vi "2d Flyover.vi"() -> ()   [LabVIEW 2022 SP3]
uses:
  C:/Users/mnopl/OneDrive/Documents/2DFlyover/2D Flyover/Thorlabs.MotionControl.Controls.dll
  Thorlabs.MotionControl.Controls.dll
  Action Engine/ActionEngineEnum.ctl
  <vilib>/DAQmx/read.llb/DAQmx Read (Analog 1D DBL 1Chan NSamp).vi
  <vilib>/Analysis/baseanly.llb/Mean (DBL).vi
  <vilib>/DAQmx/miscellaneous.llb/DAQmx Fill In Error Info.vi
  <vilib>/Analysis/NI_AALBase.lvlib
panel:
  in  "Stop":bool
  in  "Settings Y":T1={"Step Size (mm)"=10.0, "Initial Position"=0.0, "Move Absolute/Relative Position"=0.0, "Step Delay (ms)"=0, "Velocity (mm/s)"=0.0, "Acceleration (mm/s^2)"=0.0} {"Step Size (mm)" min=0.00046 format="%.8f"}
  in  "Settings X":T1={"Step Size (mm)"=10.0, "Initial Position"=0.0, "Move Absolute/Relative Position"=0.0, "Step Delay (ms)"=0, "Velocity (mm/s)"=0.0, "Acceleration (mm/s^2)"=0.0} {"Step Size (mm)" min=0.00046 format="%.8f"}
  in  "Acceleration":dbl=2.0
  in  "Estimate X Step Size":bool
  in  "2D Flyover":bool
  in  "Flyover Y Linescan":bool
  in  "Update Vel/Acc":bool
  in  "Save Line graph":bool
  out "Time Left":dbl
  out "Line Scan":dbl[](graph)
  in  "Move to Saved Pos":bool
  in  "Save Position":bool
  out "Y Pos 1":dbl
  out "X Pos 1":dbl
  in  "Save Data":bool
  in  "Move to Origin":bool
  in  "Measures/Pixel":dbl=5.0
  in  "Flyover X Linescan":bool
  in  "Move Y":bool
  in  "Move X":bool
  in  "Y Step Size":dbl=1.0
  in  "X Step Size":dbl=1.0
  in  "Move to Y":bool
  in  "Move to X":bool
  in  "Y Move":dbl=1.0
  in  "X Move":dbl=1.0
  out "Y Line Scan":dbl[](array[numeric])=[-inf, -inf, -inf, -inf, -inf, -inf]
  out "X Line Scan":dbl[](array[numeric])=[-inf, -inf, -inf, -inf, -inf, -inf]
  out "Y Origin":dbl
  out "X Orign":dbl
  out "Scan Type":string="Scan"
  in  "Y Line Scan":bool
  in  "Abort":bool
  in  "X Line Scan":bool
  out "(X,Y)":cluster{dbl, dbl}[][](array[cluster])
  in  "Save Image":bool
  in  "Move to Cursor":bool
  in  "Y Pos":dbl=0.899996795693412
  in  "X Pos":dbl=1.0
  in  "Read Position":bool
  out "Graph":dbl[][](graph)
  out "array of values":dbl[][](array[numeric])=[[-inf, -inf, -inf, -inf, -inf, -inf], [-inf, -inf, -inf, -inf, -inf, -inf], [-inf, -inf, -inf, -inf, -inf, -inf], [-inf, -inf, -inf, -inf, -inf, -inf], [-inf, -inf, -inf, -inf, -inf, -inf], [-inf, -inf, -inf, -inf, -inf, -inf]]
  out "task out":refnum<k21>
  in  "physical channels":tag="Dev3/ai0"
  in  "number of samples":i32=10000
  in  "rate":dbl=250000.0
  in  "maximum value":dbl=5.0 format="%0.2f"
  in  "minimum value":dbl=-5.0 format="%0.2f"
  out "Done Mov?":bool=TRUE
  in  "Y Length":dbl=5.0
  in  "X Length":dbl=5.0
  in  "2D Scan":bool
  in  "Velocity":dbl=2.0
  in  "Move Y (in)":bool
  in  "Move X (in)":bool
  in  "Y Step Size (in)":dbl=1.0
  in  "X Step Size (in)":dbl=1.0
  in  "X=T,Y=F":bool
  in  "Moving?":bool
  in  "KCubeStepperControl Y":refnum<k24>(container)
  in  "KCubeStepperControl X":refnum<k24>(container)
  in  "SerialNumber X":string="26005327"
  in  "SerialNumber Y":string="26005279"
  in  "Set Vel/Acc":bool
  # "Internal Variables"
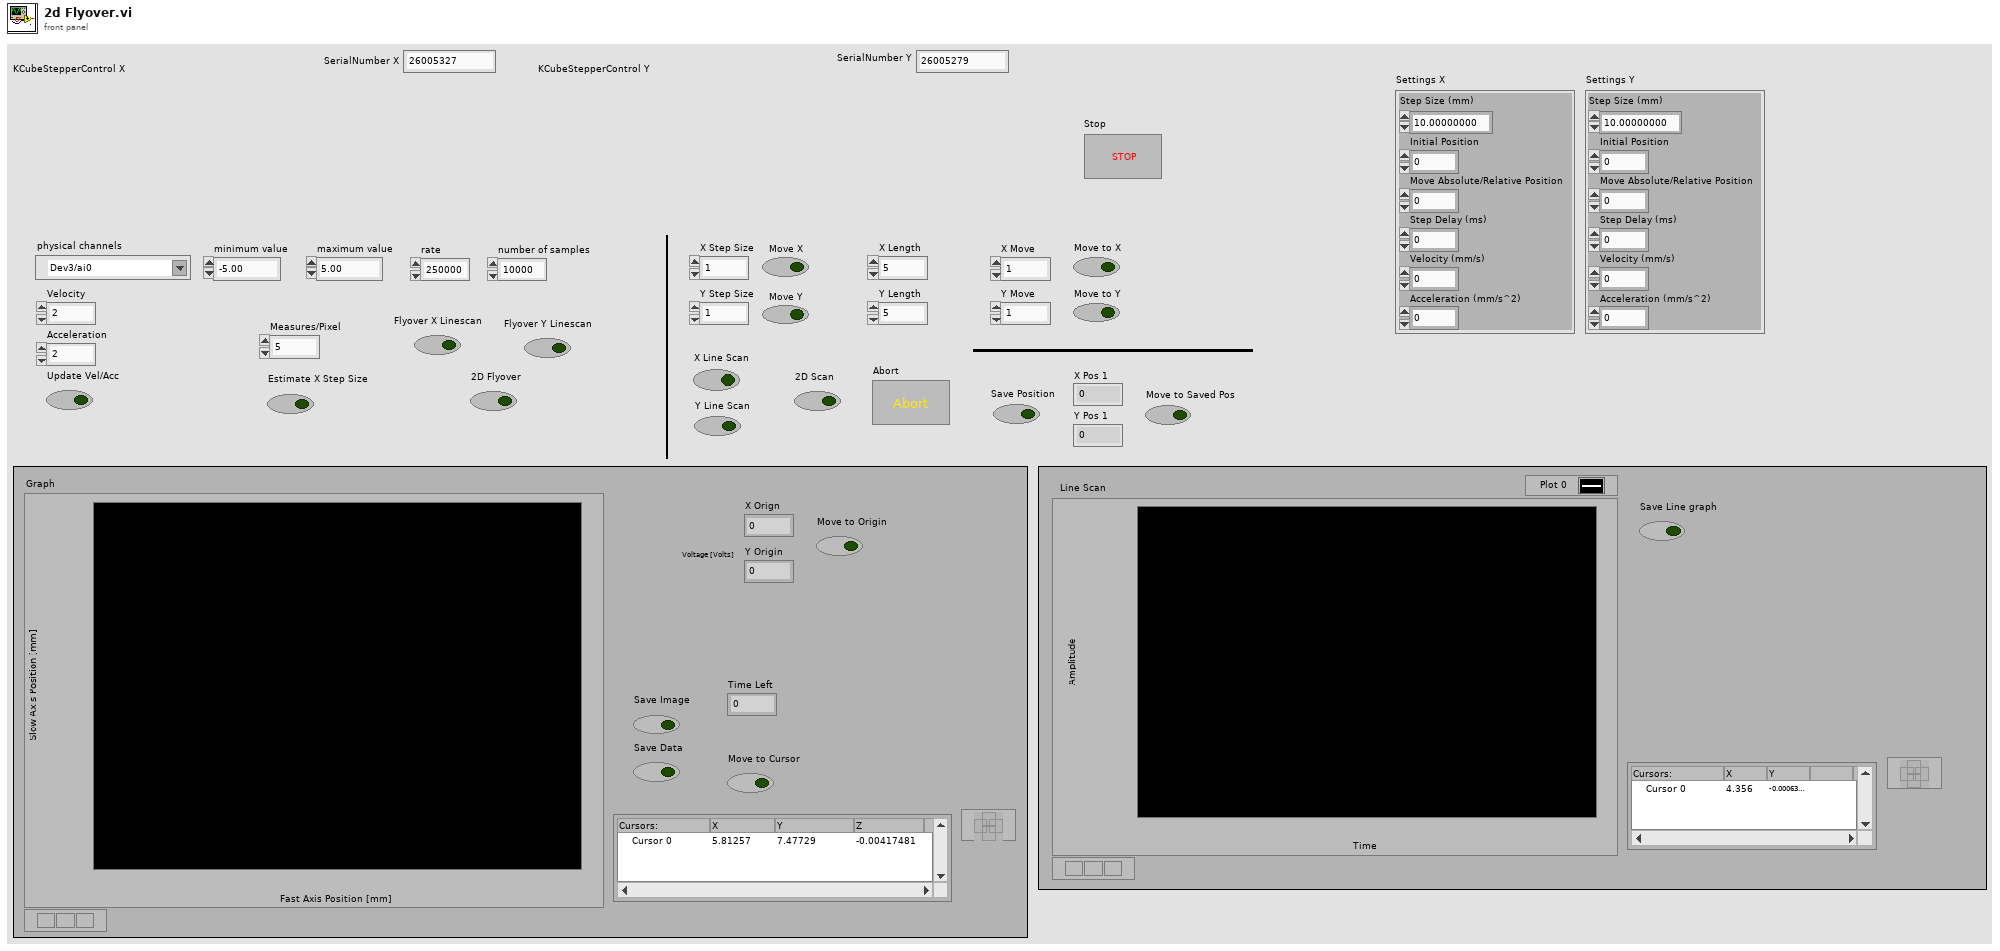
[diagram p1: front panel]
types:
  T1 = cluster{"Step Size (mm)":sgl, "Initial Position":dbl, "Move Absolute/Relative Position":dbl, "Step Delay (ms)":u32, "Velocity (mm/s)":dbl, "Acceleration (mm/s^2)":dbl}
  T2 = typedef "ActionEngineEnum.ctl" = enum16{"Open Connection", "Done", "Get Position", "Settings", "Home", "Move Absolute", "Move Relative", "Step", "Stop Action", "Close Connection"}
  T3 = typedef "LVPointDoubleTypeDef.ctl" = cluster{"Cursor X":dbl, "Cursor Y":dbl}
  T4 = typedef "imagedata.ctl" = cluster{"image type":i32, "image depth":i32, "image":u8[], "mask":u8[], "colors":u32[], "Rectangle":cluster{"left":i16, "top":i16, "right":i16, "bottom":i16}}
  T5 = cluster{"Y Step Size (in)":dbl, "Initial Position":dbl, "Move Absolute/Relative Position":dbl, "Step Delay (ms)":u32, "Velocity (mm/s)":dbl, "Acceleration (mm/s^2)":dbl}
  T6 = cluster{"X Step Size (in)":dbl, "Initial Position":dbl, "Move Absolute/Relative Position":dbl, "Step Delay (ms)":u32, "Velocity (mm/s)":dbl, "Acceleration (mm/s^2)":dbl}
  T7 = cluster{"Step Size (mm)":sgl, "Initial Position":dbl, "Move Absolute/Relative Position":dbl, "Step Delay (ms)":u32, "Velocity":dbl, "Acceleration":dbl}
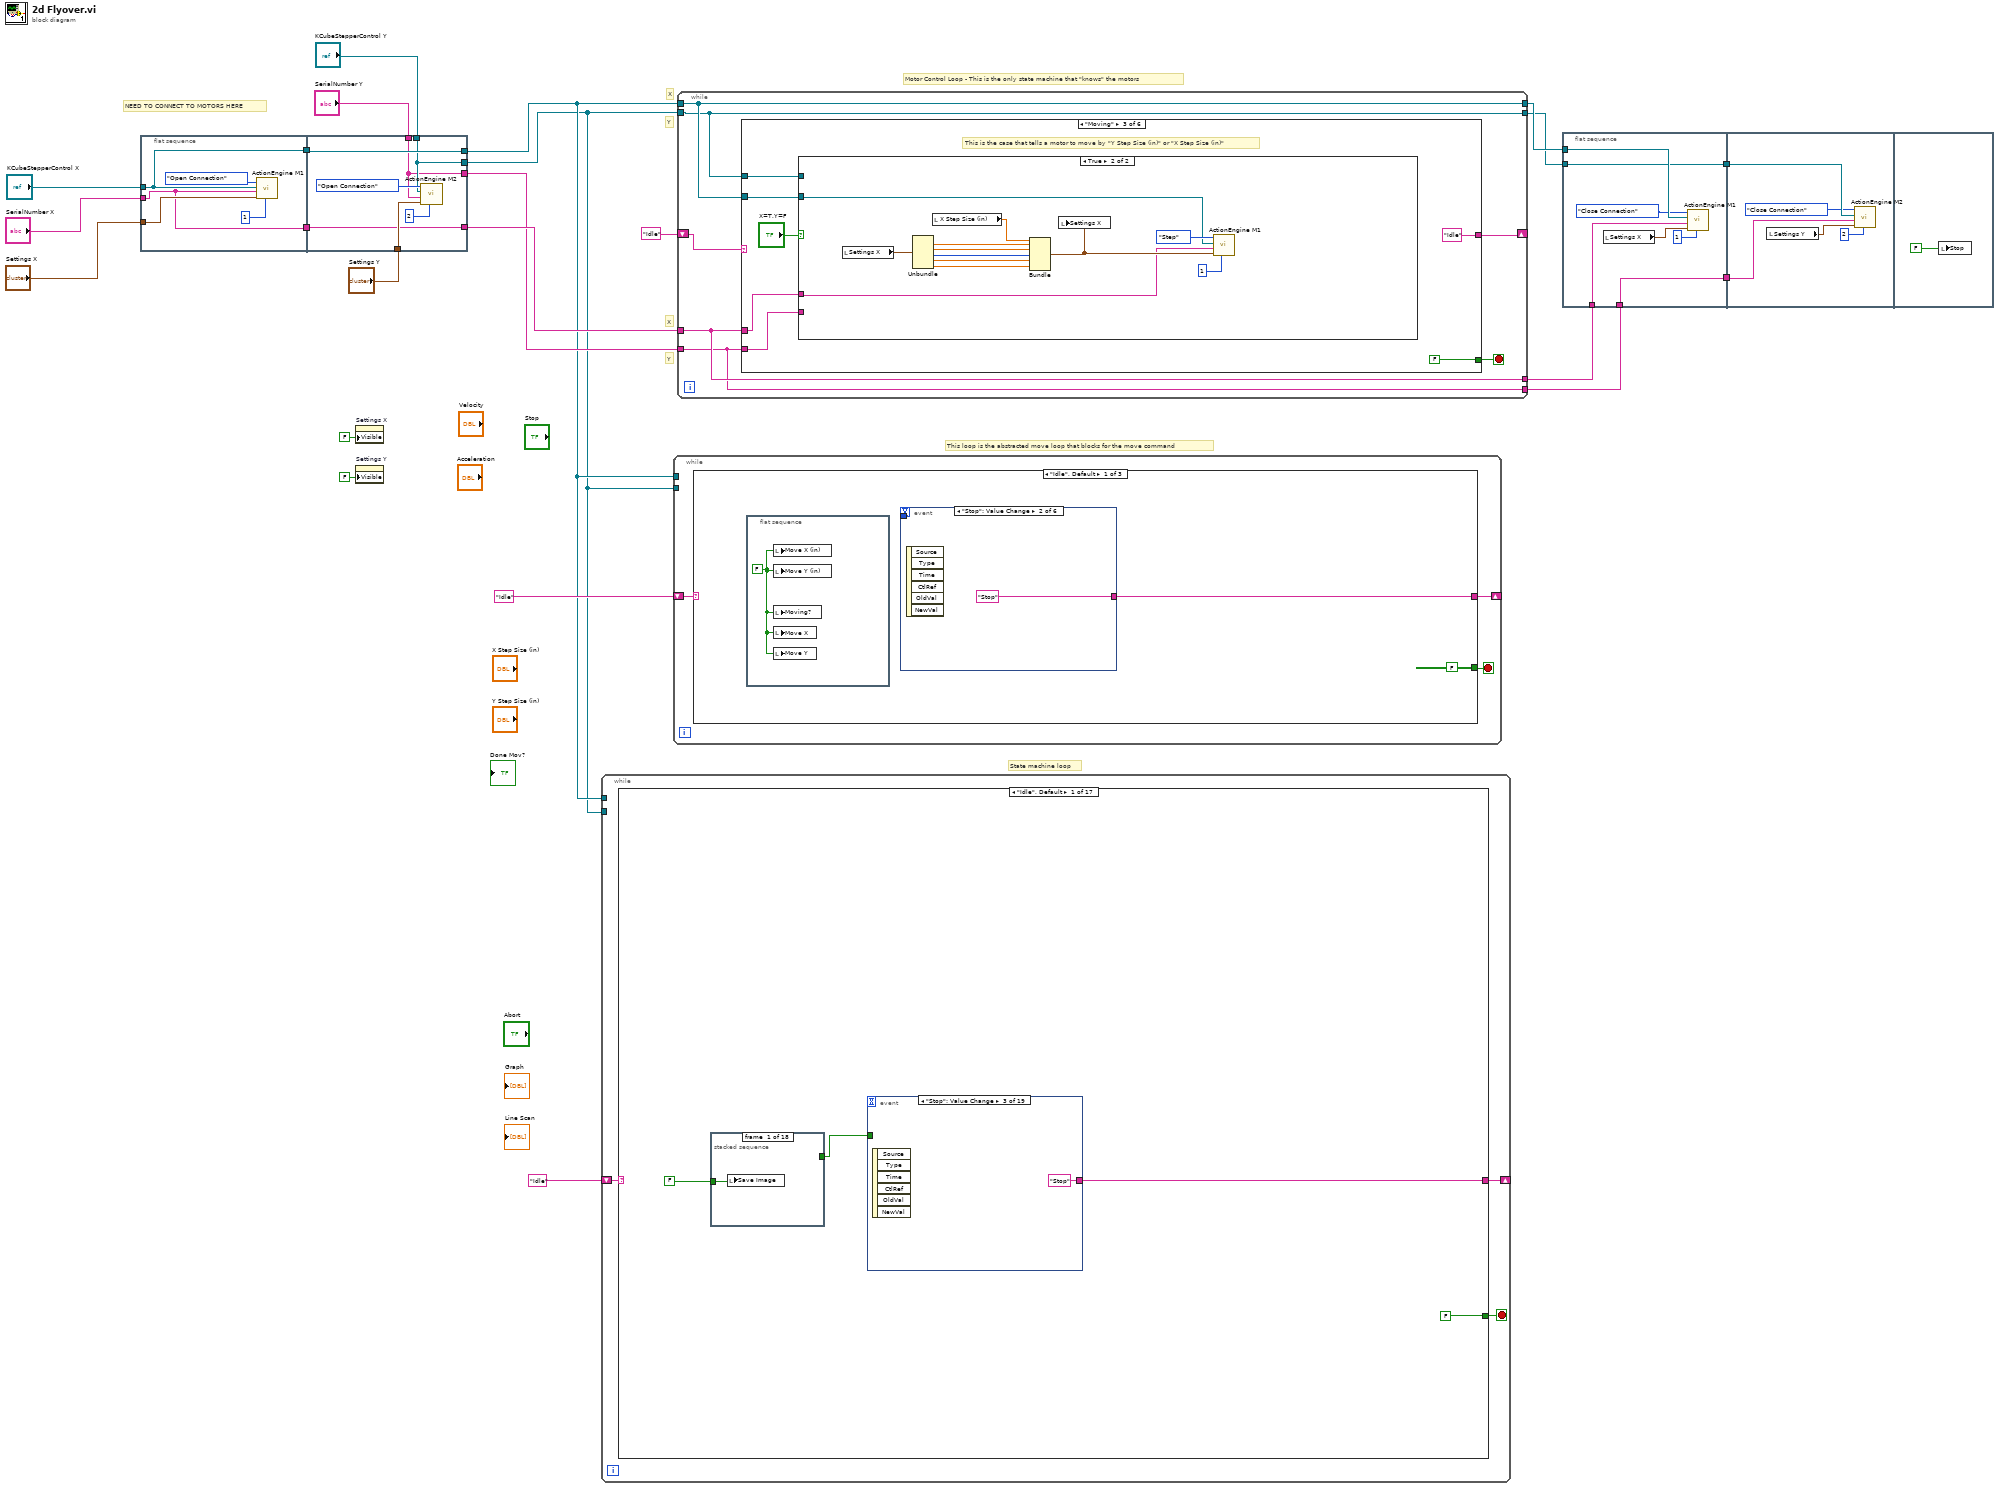
[diagram p0: block diagram]
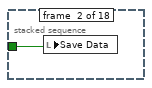
[diagram p2: hidden frame]
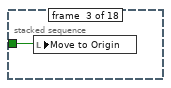
[diagram p3: hidden frame]
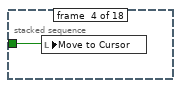
[diagram p4: hidden frame]
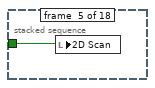
[diagram p5: hidden frame]
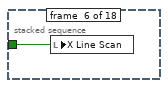
[diagram p6: hidden frame]
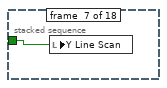
[diagram p7: hidden frame]
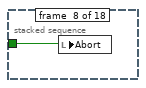
[diagram p8: hidden frame]
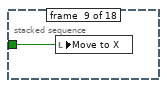
[diagram p9: hidden frame]
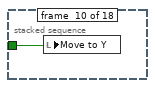
[diagram p10: hidden frame]
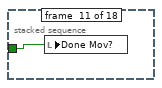
[diagram p11: hidden frame]
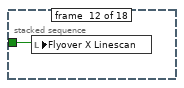
[diagram p12: hidden frame]
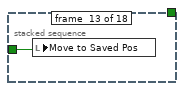
[diagram p13: hidden frame]
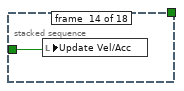
[diagram p14: hidden frame]
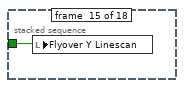
[diagram p15: hidden frame]
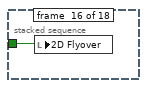
[diagram p16: hidden frame]
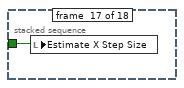
[diagram p17: hidden frame]
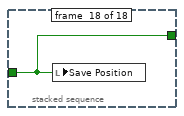
[diagram p18: hidden frame]
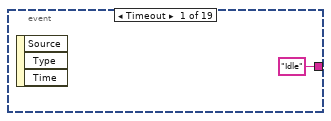
[diagram p19: hidden frame]
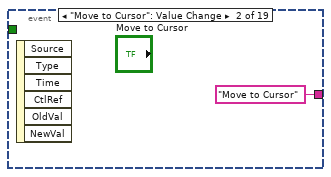
[diagram p20: hidden frame]
diagram:
  # "Y"
  # "X"
  # "NEED TO CONNECT TO MOTORS HERE"
  # "State machine loop"
  # "Y"
  # "X"
  # "This loop is the abstracted move loop that blocks for the move command"
  # "Motor Control Loop - This is the only state machine that \"knows\" the motors"
  n1 = flat-sequence {
    tunnel: "KCubeStepperControl X" -> [w25]
    tunnel: "SerialNumber X" -> [w24]
    tunnel: "Settings X" -> [w26]
    tunnel: [w25] -> w14
    tunnel: [w24] -> w13
    tunnel: "KCubeStepperControl Y" -> [w31]
    tunnel: "SerialNumber Y" -> [w29]
    tunnel: "Settings Y" -> [w33]
    tunnel: w14 -> [w32]
    tunnel: [w32] -> w10
    tunnel: [w31] -> w9
    tunnel: w13 -> [w30]
    tunnel: [w30] -> w12
    tunnel: [w29] -> w11
    frame #0 {
      n2 = call "ActionEngine M1.vi"("ChannelNumber"=1, "Settings"=w26, "SerialNumber"=w24, "KCubeStepperControl"=w25, "Action"=ActionEngineEnum."Open Connection") -> ()  [unwired: 4 in, 2 out]
    }
    frame #1 {
      n3 = call "ActionEngine M2.vi"("ChannelNumber"=2, "Settings"=w33, "SerialNumber"=w29, "KCubeStepperControl"=w31, "Action"=ActionEngineEnum."Open Connection") -> ()  [unwired: 4 in, 2 out]
    }
  }
  n4 = property on="Settings X" class="Clust (strict)"("Visible"=FALSE) -> ()  [unwired: 2 in, 2 out]
  n5 = property on="Settings Y" class="Clust (strict)"("Visible"=FALSE) -> ()  [unwired: 2 in, 2 out]
  n6 = while {
    shift-right: [w37] -> _
    shift-left: "Idle" -> [w38]
    tunnel: w10 -> [_]
    tunnel: w9 -> [_]
    stop <- w36 stop-if-true
    n7 = case shown="\"Idle\", Default" w38 {
      tunnel: [w42 "Init Graph" w132 "Move to Origin" w471 "Idle" ("Scan Type") "Move to Origin" ("Scan Type") "Move to Origin" ("Scan Type") "Idle" ("Scan Type") "Idle" ("Scan Type") "Idle" "Idle" ("Scan Type") "Idle" ("Scan Type") "Idle" ("Scan Type") "Idle" "Idle" ("Scan Type") "Idle"] -> w37
      tunnel: [FALSE FALSE FALSE FALSE FALSE FALSE FALSE FALSE FALSE FALSE FALSE FALSE FALSE FALSE FALSE FALSE TRUE] -> w36
      frame "Idle", Default {
        n8 = stacked-sequence {
          tunnel: FALSE -> [w43 w44 w45 w46 w47 w48 w49 w50 w51 w52 w53 w54 w55 w56 w57 w58 w59 w60]
          tunnel: [_ _ _ _ _ _ _ _ _ _ _ _ _ _ _ _ _ w60] -> w39
          frame #0 {
            n9 = local write "Save Image"(w43) -> ()
          }
          frame #1 {
            n10 = local write "Save Data"(w44) -> ()
          }
          frame #2 {
            n11 = local write "Move to Origin"(w45) -> ()
          }
          frame #3 {
            n12 = local write "Move to Cursor"(w46) -> ()
          }
          frame #4 {
            n13 = local write "2D Scan"(w47) -> ()
          }
          frame #5 {
            n14 = local write "X Line Scan"(w48) -> ()
          }
          frame #6 {
            n15 = local write "Y Line Scan"(w49) -> ()
          }
          frame #7 {
            n16 = local write "Abort"(w50) -> ()
          }
          frame #8 {
            n17 = local write "Move to X"(w51) -> ()
          }
          frame #9 {
            n18 = local write "Move to Y"(w52) -> ()
          }
          frame #10 {
            n19 = local write "Done Mov?"(w53) -> ()
          }
          frame #11 {
            n20 = local write "Flyover X Linescan"(w54) -> ()
          }
          frame #12 {
            n21 = local write "Move to Saved Pos"(w55) -> ()
          }
          frame #13 {
            n22 = local write "Update Vel/Acc"(w56) -> ()
          }
          frame #14 {
            n23 = local write "Flyover Y Linescan"(w57) -> ()
          }
          frame #15 {
            n24 = local write "2D Flyover"(w58) -> ()
          }
          frame #16 {
            n25 = local write "Estimate X Step Size"(w59) -> ()
          }
          frame #17 {
            n26 = local write "Save Position"(w60) -> ()
          }
        }
        n27 = event shown="[2] \"Stop\": Value Change" {
          selector: _ -> [_ _ _ _ _ _ _ _ _ _ _ _ _ _ _ _ _ _ _]
          dyn-events: _ -> [_ _ _ _ _ _ _ _ _ _ _ _ _ _ _ _ _ _ _]
          timeout: _ -> [_ _ _ _ _ _ _ _ _ _ _ _ _ _ _ _ _ _ _]
          tunnel: ["Idle" "Move to Cursor" "Stop" "Init Daq" "Init Daq" "Move to Origin" "Move to Saved Position" "Init Daq" "Init Daq" "Init Daq" "Init Daq" "Move to" "Move to" "Update Vel/Acc" "Save Position" "Save Image" "Save Line graph" "Save Data" "Estimate X Step Size"] -> w42
          tunnel: w39 -> [_ _ _ _ _ _ _ _ _ _ _ _ _ _ _ _ _ _ _]
          event Timeout {
            n28 = event-data() -> ()  [unwired: 1 in, 3 out]
          }
          event "Move to Cursor": Value Change {
            n29 = event-data() -> ()  [unwired: 1 in, 6 out]
          }
          event "Stop": Value Change {
            n30 = event-data() -> ()  [unwired: 1 in, 6 out]
          }
          event "2D Scan": Value Change {
            n31 = event-data() -> ()  [unwired: 1 in, 6 out]
            n32 = local read "X Step Size"() -> (w64:dbl)
            n33 = local read "Y Step Size"() -> (w65:dbl)
            n34 = local write "Scan Type"("Scan" ("Scan Type")) -> ()
            n35 = local write "Y Step Size (in)"(w65) -> ()
            n36 = local write "X Step Size (in)"(w64) -> ()
          }
          event "2D Flyover": Value Change {
            n37 = event-data() -> ()  [unwired: 1 in, 6 out]
            n38 = local read "Y Step Size"() -> (w69:dbl)
            n39 = local read "X Step Size"() -> (w70:dbl)
            n40 = local write "X Step Size (in)"(w70) -> ()
            n41 = local write "Y Step Size (in)"(w69) -> ()
            n42 = local write "Scan Type"("Flyover Scan" ("Scan Type")) -> ()
          }
          event "Move to Origin": Value Change {
            n43 = event-data() -> ()  [unwired: 1 in, 6 out]
          }
          event "Move to Saved Pos": Value Change {
            n44 = event-data() -> ()  [unwired: 1 in, 6 out]
          }
          event "X Line Scan": Value Change {
            n45 = event-data() -> ()  [unwired: 1 in, 6 out]
            n46 = local read "X Step Size"() -> (w74:dbl)
            n47 = local write "X Step Size (in)"(w74) -> ()
            n48 = local write "Scan Type"("Line Scan" ("Scan Type")) -> ()
            n49 = local write "X=T,Y=F"(TRUE ("X=T,Y=F")) -> ()
          }
          event "Flyover X Linescan": Value Change {
            n50 = event-data() -> ()  [unwired: 1 in, 6 out]
            n51 = local read "X Step Size"() -> (w81:dbl)
            n52 = local write "X Step Size (in)"(w81) -> ()
            n53 = local write "Scan Type"("Flyover Linescan" ("Scan Type")) -> ()
            n54 = local write "X=T,Y=F"(TRUE ("X=T,Y=F")) -> ()
          }
          event "Flyover Y Linescan": Value Change {
            n55 = event-data() -> ()  [unwired: 1 in, 6 out]
            n56 = local read "Y Step Size"() -> (w83:dbl)
            n57 = local write "Y Step Size (in)"(w83) -> ()
            n58 = local write "Scan Type"("Flyover Linescan" ("Scan Type")) -> ()
            n59 = local write "X=T,Y=F"(FALSE ("X=T,Y=F")) -> ()
          }
          event "Y Line Scan": Value Change {
            n60 = event-data() -> ()  [unwired: 1 in, 6 out]
            n61 = local read "Y Step Size"() -> (w86:dbl)
            n62 = local write "Y Step Size (in)"(w86) -> ()
            n63 = local write "X=T,Y=F"(FALSE ("X=T,Y=F")) -> ()
            "Scan Type" <- "Line Scan" ("Scan Type")
          }
          event "Move to X": Value Change {
            n64 = event-data() -> ()  [unwired: 1 in, 6 out]
            n65 = local write "X=T,Y=F"(TRUE ("X=T,Y=F")) -> ()
          }
          event "Move to Y": Value Change {
            n66 = event-data() -> ()  [unwired: 1 in, 6 out]
            n67 = local write "X=T,Y=F"(FALSE ("X=T,Y=F")) -> ()
          }
          event "Update Vel/Acc": Value Change {
            n68 = event-data() -> ()  [unwired: 1 in, 6 out]
          }
          event "Save Position": Value Change {
            n69 = event-data() -> ()  [unwired: 1 in, 6 out]
          }
          event "Save Image": Value Change {
            n70 = event-data() -> ()  [unwired: 1 in, 6 out]
          }
          event "Save Line graph": Value Change {
            n71 = event-data() -> ()  [unwired: 1 in, 6 out]
          }
          event "Save Data": Value Change {
            n72 = event-data() -> ()  [unwired: 1 in, 6 out]
          }
          event "Estimate X Step Size": Value Change {
            n73 = event-data() -> ()  [unwired: 1 in, 6 out]
          }
        }
      }
      frame "Init Daq" {
        w100 = -inf
        n74 = local read "Y Length"() -> (w113:dbl)
        n75 = local read "Y Step Size"() -> (w112:dbl)
        n76 = local read "X Length"() -> (w110:dbl)
        n77 = local read "X Step Size"() -> (w109:dbl)
        n78 = Divide(x=w113, y=w112) -> (x/y=w114:dbl)
        n79 = Divide(x=w110, y=w109) -> (x/y=w111:dbl)
        n80 = Round Toward +Infinity(x=w114) -> (ceil(x): smallest int >= x=w103:dbl)
        n81 = Round Toward +Infinity(x=w111) -> (ceil(x): smallest int >= x=w108:dbl)
        n82 = Increment(x=w103) -> (x+1=w101:dbl)
        n83 = Increment(x=w108) -> (x+1=w102:dbl)
        n84 = call "Initialize DAQ Assistant.vi"("minimum value"="minimum value", "maximum value"="maximum value", "rate"="rate", "number of samples"="number of samples", "physical channels"="physical channels") -> ("task out"=→"task out":refnum<k21>)  [unwired: 5 in, 1 out]
        n85 = Initialize Array(w100, w101) -> (→"Y Line Scan":dbl[])
        n86 = Initialize Array(w100, w102, w101) -> (→"array of values":dbl[][])
        n87 = Initialize Array(w100, w102) -> (→"X Line Scan":dbl[])
      }
      frame "Init Graph" {
        n88 = local read "Acceleration"() -> (w128:dbl)
        n89 = local read "Scan Type"() -> (w132:string)
        n90 = local read "Velocity"() -> (w129:dbl)
        n91 = flat-sequence {
          tunnel: [w201] -> w122
          tunnel: ["X Pos"] -> w134
          tunnel: ["Y Pos"] -> w133
          frame #0 {
            n92 = property on="Read Position" class="Bool (strict)"("Val(Sgnl)"=TRUE) -> ()  [unwired: 2 in, 2 out]
          }
          frame #1 {
            n93 = while {
              tunnel: [w202] -> w201
              stop <- w205 stop-if-true
              n94 = local read "Read Position"() -> (w204:bool)
              n95 = Not(x=w204) -> (.not. x?=w205:bool)
              n96 = Wait (ms)(milliseconds to wait=u32 10) -> (millisecond timer value=w202:u32)
            }
          }
          frame #2 {
            "X Orign" <- "X Pos"
            "Y Origin" <- "Y Pos"
          }
        }
        n97 = case shown="\"Line Scan\", Default" w132 {
          tunnel: [w150 w168 w184] -> w126
          tunnel: w125 -> [w150 w168 w184]
          frame "Line Scan", Default {
            n98 = local read "X=T,Y=F"() -> (w151:bool)
            n99 = case shown="True" w151 {
              frame False {
                n100 = flat-sequence {
                  frame #0 {
                    n101 = local read "Y Length"() -> (w153:dbl)
                    n102 = Divide(x=w153, y=2.0) -> (x/y=w154:dbl)
                    n103 = Negate(x=w154) -> (-x=w155:dbl)
                    n104 = local write "Y Step Size (in)"(w155) -> ()
                  }
                  frame #1 {
                    n105 = local write "Done Mov?"(FALSE ("Done Mov?")) -> ()
                    n106 = property on="Move Y (in)" class="Bool (strict)"("Val(Sgnl)"=TRUE ("Value (Signaling)")) -> ()  [unwired: 2 in, 2 out]
                  }
                  frame #2 {
                    n107 = while {
                      stop <- w158 stop-if-true
                      n108 = local read "Done Mov?"() -> (w158:bool)
                    }
                  }
                  frame #3 {
                    n109 = local write "Done Mov?"(FALSE ("Done Mov?")) -> ()
                  }
                }
              }
              frame True {
                n110 = flat-sequence {
                  frame #0 {
                    n111 = local read "X Length"() -> (w163:dbl)
                    n112 = Divide(x=w163, y=2.0) -> (x/y=w162:dbl)
                    n113 = Negate(x=w162) -> (-x=w161:dbl)
                    n114 = local write "X Step Size (in)"(w161) -> ()
                  }
                  frame #1 {
                    n115 = property on="Move X (in)" class="Bool (strict)"("Val(Sgnl)"=TRUE ("Value (Signaling)")) -> ()  [unwired: 2 in, 2 out]
                    n116 = local write "Done Mov?"(FALSE ("Done Mov?")) -> ()
                  }
                  frame #2 {
                    n117 = while {
                      stop <- w166 stop-if-true
                      n118 = local read "Done Mov?"() -> (w166:bool)
                    }
                  }
                  frame #3 {
                    n119 = local write "Done Mov?"(FALSE ("Done Mov?")) -> ()
                  }
                }
              }
            }
          }
          frame "Scan" {
            n120 = flat-sequence {
              frame #0 {
                n121 = local read "X Length"() -> (w176:dbl)
                n122 = local read "Y Length"() -> (w174:dbl)
                n123 = Divide(x=w176, y=2.0) -> (x/y=w172:dbl)
                n124 = Divide(x=w174, y=2.0) -> (x/y=w170:dbl)
                n125 = Negate(x=w172) -> (-x=w171:dbl)
                n126 = Negate(x=w170) -> (-x=w169:dbl)
                n127 = local write "X Step Size (in)"(w171) -> ()
                n128 = local write "Y Step Size (in)"(w169) -> ()
              }
              frame #1 {
                n129 = local write "Done Mov?"(FALSE ("Done Mov?")) -> ()
                n130 = property on="Move Y (in)" class="Bool (strict)"("Val(Sgnl)"=TRUE ("Value (Signaling)")) -> ()  [unwired: 2 in, 2 out]
              }
              frame #2 {
                n131 = while {
                  stop <- w179 stop-if-true
                  n132 = local read "Done Mov?"() -> (w179:bool)
                }
              }
              frame #3 {
                n133 = local write "Done Mov?"(FALSE ("Done Mov?")) -> ()
                n134 = property on="Move X (in)" class="Bool (strict)"("Val(Sgnl)"=TRUE ("Value (Signaling)")) -> ()  [unwired: 2 in, 2 out]
              }
              frame #4 {
                n135 = while {
                  stop <- w182 stop-if-true
                  n136 = local read "Done Mov?"() -> (w182:bool)
                }
              }
              frame #5 {
                n137 = local write "Done Mov?"(FALSE ("Done Mov?")) -> ()
              }
            }
          }
          frame "Flyover Scan" {
            n138 = flat-sequence {
              frame #0 {
                n139 = local read "X Length"() -> (w192:dbl)
                n140 = local read "Y Length"() -> (w190:dbl)
                n141 = Divide(x=w192, y=2.0) -> (x/y=w188:dbl)
                n142 = Divide(x=w190, y=2.0) -> (x/y=w186:dbl)
                n143 = Negate(x=w188) -> (-x=w187:dbl)
                n144 = Negate(x=w186) -> (-x=w185:dbl)
                n145 = local write "X Step Size (in)"(w187) -> ()
                n146 = local write "Y Step Size (in)"(w185) -> ()
              }
              frame #1 {
                n147 = local write "Done Mov?"(FALSE ("Done Mov?")) -> ()
                n148 = property on="Move Y (in)" class="Bool (strict)"("Val(Sgnl)"=TRUE ("Value (Signaling)")) -> ()  [unwired: 2 in, 2 out]
              }
              frame #2 {
                n149 = while {
                  stop <- w195 stop-if-true
                  n150 = local read "Done Mov?"() -> (w195:bool)
                }
              }
              frame #3 {
                n151 = local write "Done Mov?"(FALSE ("Done Mov?")) -> ()
                n152 = property on="Move X (in)" class="Bool (strict)"("Val(Sgnl)"=TRUE ("Value (Signaling)")) -> ()  [unwired: 2 in, 2 out]
              }
              frame #4 {
                n153 = while {
                  stop <- w198 stop-if-true
                  n154 = local read "Done Mov?"() -> (w198:bool)
                }
              }
              frame #5 {
                n155 = local write "Done Mov?"(FALSE ("Done Mov?")) -> ()
              }
            }
          }
        }
        n156 = flat-sequence {
          tunnel: w129 -> [w139]
          tunnel: [w139] -> w131
          tunnel: w128 -> [w136]
          tunnel: [w136] -> w130
          tunnel: w122 -> [_]
          tunnel: w131 -> [w142]
          tunnel: w130 -> [w141]
          tunnel: [w142] -> w124
          tunnel: [w141] -> w123
          tunnel: [w144] -> w125
          tunnel: [w145] -> w127
          tunnel: w124 -> [w145]
          tunnel: w123 -> [w144]
          frame #0 {
            n157 = local write "Acceleration"(10.0 ("Acceleration")) -> ()
            n158 = local write "Velocity"(2.0 ("Velocity")) -> ()
          }
          frame #1 {
            n159 = property on="Set Vel/Acc" class="Bool (strict)"("Val(Sgnl)"=TRUE ("Value (Signaling)")) -> ()  [unwired: 2 in, 2 out]
          }
          frame #2 {
            n160 = Wait (ms)(milliseconds to wait=u32 150) -> ()  [unwired: 1 out]
          }
        }
        n161 = case shown="\"Line Scan\", Default" w132 {
          tunnel: w134 -> [w211 w230 w242]
          tunnel: w133 -> [w210 w225 w237]
          frame "Line Scan", Default {
            n162 = local read "X=T,Y=F"() -> (w209:bool)
            n163 = case shown="False" w209 {
              tunnel: w211 -> [_ w223]
              tunnel: w210 -> [w217 _]
              tunnel: [w212 w218] -> w208
              frame False {
                n164 = local read "Y Length"() -> (w215:dbl)
                n165 = local read "Y Step Size"() -> (w212:dbl)
                n166 = Divide(x=w215, y=2.0) -> (x/y=w213:dbl)
                n167 = Subtract(x=w217, y=w213) -> (x-y=w216:dbl)
                n168 = property on="Line Scan" class="WFGraph (strict)"("XScale.Offset"=w216) -> ()  [unwired: 2 in, 2 out]
              }
              frame True {
                n169 = local read "X Length"() -> (w221:dbl)
                n170 = Divide(x=w221, y=2.0) -> (x/y=w219:dbl)
                n171 = Subtract(x=w223, y=w219) -> (x-y=w222:dbl)
                n172 = local read "X Step Size"() -> (w218:dbl)
                n173 = property on="Line Scan" class="WFGraph (strict)"("XScale.Offset"=w222) -> ()  [unwired: 2 in, 2 out]
              }
            }
            n174 = property on="Line Scan" class="WFGraph (strict)"("XScale.Multiplier"=w208) -> ()  [unwired: 2 in, 2 out]
          }
          frame "Scan" {
            n175 = local read "X Length"() -> (w233:dbl)
            n176 = local read "Y Length"() -> (w228:dbl)
            n177 = Divide(x=w233, y=2.0) -> (x/y=w231:dbl)
            n178 = Divide(x=w228, y=2.0) -> (x/y=w226:dbl)
            n179 = local read "Y Step Size"() -> (w235:dbl)
            n180 = local read "X Step Size"() -> (w234:dbl)
            n181 = Subtract(x=w225, y=w226) -> (x-y=w224:dbl)
            n182 = Subtract(x=w230, y=w231) -> (x-y=w229:dbl)
            n183 = property on="Graph" class="IntGraph (strict)"("XScale.Offset"=w229) -> ()  [unwired: 2 in, 2 out]
            n184 = property on="Graph" class="IntGraph (strict)"("YScale.Offset"=w224) -> ()  [unwired: 2 in, 2 out]
            n185 = property on="Graph" class="IntGraph (strict)"("YScale.Multiplier"=w235) -> ()  [unwired: 2 in, 2 out]
            n186 = property on="Graph" class="IntGraph (strict)"("XScale.Multiplier"=w234) -> ()  [unwired: 2 in, 2 out]
          }
          frame "Flyover Scan" {
            n187 = local read "X Length"() -> (w245:dbl)
            n188 = local read "Y Length"() -> (w240:dbl)
            n189 = Divide(x=w245, y=2.0) -> (x/y=w243:dbl)
            n190 = Divide(x=w240, y=2.0) -> (x/y=w238:dbl)
            n191 = local read "Y Step Size"() -> (w247:dbl)
            n192 = local read "X Step Size"() -> (w246:dbl)
            n193 = Subtract(x=w237, y=w238) -> (x-y=w236:dbl)
            n194 = Subtract(x=w242, y=w243) -> (x-y=w241:dbl)
            n195 = property on="Graph" class="IntGraph (strict)"("XScale.Offset"=w241) -> ()  [unwired: 2 in, 2 out]
            n196 = property on="Graph" class="IntGraph (strict)"("YScale.Offset"=w236) -> ()  [unwired: 2 in, 2 out]
            n197 = property on="Graph" class="IntGraph (strict)"("YScale.Multiplier"=w247) -> ()  [unwired: 2 in, 2 out]
            n198 = property on="Graph" class="IntGraph (strict)"("XScale.Multiplier"=w246) -> ()  [unwired: 2 in, 2 out]
          }
        }
        n199 = flat-sequence {
          tunnel: w126 -> [w147]
          tunnel: w127 -> [w146]
          frame #0 {
            n200 = local write "Velocity"(w146) -> ()
            n201 = local write "Acceleration"(w147) -> ()
          }
          frame #1 {
            n202 = property on="Set Vel/Acc" class="Bool (strict)"("Val(Sgnl)"=TRUE ("Value (Signaling)")) -> ()  [unwired: 2 in, 2 out]
          }
          frame #2 {
            n203 = Wait (ms)(milliseconds to wait=u32 150) -> ()  [unwired: 1 out]
          }
        }
      }
      frame "Scan" {
        w255 = 0 ("Row")
        n204 = local read "number of samples"() -> (w251:i32)
        n205 = local read "Y Step Size"() -> (w249:dbl)
        n206 = local read "array of values"() -> (w253:dbl[][])
        n207 = local read "Y Origin"() -> (w260:dbl)
        n208 = local read "task out"() -> (w254:refnum<k21>)
        n209 = local read "X Orign"() -> (w262:dbl)
        n210 = local read "X Step Size"() -> (w266:dbl)
        n211 = Divide(x="Y Length", y=2.0) -> (x/y=w258:dbl)
        n212 = Divide(x="X Length", y=2.0) -> (x/y=w261:dbl)
        n213 = Divide(x="Y Length", y=w249) -> (x/y=w248:dbl)
        n214 = call "Measure and Update Array.vi"("Array In"=w253, "number of samples per channel"=w251, "task/channels in"=w254, "Row"=w255, "Column"=w255) -> ("Array Out"=w252:dbl[][])  [unwired: 7 in, 3 out]
        n215 = local write "Graph"(w252) -> ()
        n216 = Subtract(x=w260, y=w258) -> (x-y=w256:dbl)
        n217 = Subtract(x=w262, y=w261) -> (x-y=w257:dbl)
        n218 = while {
          shift-right: [w301] -> w268
          shift-left: w252 -> [w302]
          tunnel: [w297] -> w267 mode=indexing
          tunnel: "X Length" -> [w293]
          tunnel: w266 -> [w296]
          tunnel: w249 -> [w295]
          tunnel: "Y Length" -> [w294]
          tunnel: [w289] -> w265
          tunnel: "X Length" -> [w292]
          tunnel: w257 -> [w288]
          tunnel: w256 -> [w287]
          tunnel: w248 -> [w282]
          i -> [w299]
          stop <- w304 stop-if-true
          n219 = Multiply(x=w299, y=w295) -> (x*y=w298:dbl)
          n220 = while {
            tunnel: [w413] -> w291
            tunnel: w299 -> [w413]
            tunnel: [w412] -> w303
            shift-right: [w408] -> w275
            shift-left: w302 -> [w411]
            tunnel: [w410] -> w290
            tunnel: [w409] -> w300
            tunnel: w298 -> [w399]
            tunnel: [w407] -> w297 mode=indexing
            tunnel: w293 -> [w405]
            tunnel: w296 -> [w406]
            tunnel: w288 -> [w398]
            tunnel: w287 -> [w396]
            tunnel: [w394] -> w274
            i -> [w420]
            stop <- w417 stop-if-true
            n221 = flat-sequence {
              tunnel: w406 -> [w421]
              tunnel: w405 -> [w422]
              tunnel: w420 -> [w423]
              tunnel: [w423] -> w404
              tunnel: [w422] -> w403
              tunnel: [w421] -> w402
              tunnel: [w421] -> w395
              tunnel: [w433] -> w419
              tunnel: [w428] -> w414
              tunnel: [w424] -> w400
              tunnel: w404 -> [w426]
              tunnel: w403 -> [w430]
              tunnel: w402 -> [w429]
              tunnel: w395 -> [w425]
              tunnel: w419 -> [w436]
              tunnel: [w437] -> w418
              tunnel: [w439] -> w416
              tunnel: [w438] -> w415
              tunnel: w414 -> [w438]
              tunnel: [w434] -> w394
              tunnel: [w450] -> w417
              tunnel: w418 -> [w450]
              tunnel: w416 -> [_]
              tunnel: w415 -> [w443]
              tunnel: w413 -> [w448]
              tunnel: [w443] -> w412
              tunnel: [w447] -> w408
              tunnel: w411 -> [w446]
              tunnel: [w445] -> w410
              tunnel: [w444] -> w409
              frame #0 {
                n222 = local write "X Step Size (in)"(w421) -> ()
              }
              frame #1 {
                n223 = Increment(x=w426) -> (x+1=w428:i32)
                n224 = Multiply(x=w426, y=w425) -> (x*y=w424:dbl)
                n225 = local write "Done Mov?"(FALSE ("Done Moving?")) -> ()
                n226 = property on="Move X (in)" class="Bool (strict)"("Val(Sgnl)"=TRUE) -> ()  [unwired: 2 in, 2 out]
                n227 = Multiply(x=w429, y=w428) -> (x*y=w432:dbl)
                n228 = Less Or Equal?(x=w430, y=w432) -> (x <= y?=w433:bool)
              }
              frame #2 {
                n229 = while {
                  tunnel: [w441] -> w439
                  tunnel: [w440] -> w435
                  tunnel: [w440] -> w434
                  stop <- w442 stop-if-true
                  n230 = local read "Done Mov?"() -> (w441:bool)
                  n231 = local read "Abort"() -> (w440:bool)
                  n232 = Or(x=w441, y=w440) -> (x .or. y?=w442:bool)
                }
                n233 = Or(x=w436, y=w435) -> (x .or. y?=w437:bool)
              }
              frame #3 {
                n234 = local read "number of samples"() -> (w445:i32)
                n235 = local read "task out"() -> (w449:refnum<k21>)
                n236 = call "Measure and Update Array.vi"("Array In"=w446, "number of samples per channel"=w445, "task/channels in"=w449, "Row"=w443, "Column"=w448) -> ("Array Out"=w447:dbl[][], "task out"=w444:refnum<k21>)  [unwired: 7 in, 2 out]
              }
            }
            n237 = Add(x=w396, y=w399) -> (x+y=w397:dbl)
            n238 = Add(x=w400, y=w398) -> (x+y=w401:dbl)
            n239 = Bundle(w401, w397) -> (w407:cluster{dbl, dbl})  [unwired: 1 in]
            n240 = local write "Graph"(w408) -> ()
          }
          n241 = case shown="False" w274 {
            tunnel: [w318 TRUE] -> w304
            tunnel: w303 -> [w317 _]
            tunnel: [w316 w392] -> w301
            tunnel: w300 -> [w315 w391]
            tunnel: w295 -> [w314 _]
            tunnel: [w313 w391] -> w289
            tunnel: w294 -> [w312 _]
            tunnel: w292 -> [w311 _]
            tunnel: w291 -> [w310 _]
            tunnel: w275 -> [w309 w392]
            tunnel: w290 -> [w308 _]
            tunnel: [w306 w390] -> w285
            tunnel: [w305 1.0] -> w279
            frame False {
              n242 = flat-sequence {
                tunnel: w312 -> [w340]
                tunnel: w314 -> [w335]
                tunnel: w310 -> [w341]
                tunnel: [w341] -> w334
                tunnel: [w335] -> w333
                tunnel: [w340] -> w332
                tunnel: w311 -> [w339]
                tunnel: [TRUE ("Value (Signaling)")] -> w331
                tunnel: [w346] -> w330
                tunnel: [w345] -> w329
                tunnel: [w344] -> w328
                tunnel: w334 -> [w346]
                tunnel: w333 -> [w345]
                tunnel: w332 -> [w344]
                tunnel: w331 -> [w343]
                tunnel: [w342] -> w307
                tunnel: [w351] -> w327
                tunnel: [w349] -> w326
                tunnel: [w350] -> w325
                tunnel: w330 -> [w351]
                tunnel: w329 -> [w349]
                tunnel: w328 -> [w350]
                tunnel: [w348] -> w324
                tunnel: w307 -> [w347]
                tunnel: [w363] -> w323
                tunnel: [w358] -> w322
                tunnel: w327 -> [w359]
                tunnel: w326 -> [w361]
                tunnel: w325 -> [w356]
                tunnel: w324 -> [_]
                tunnel: [w355] -> w305
                tunnel: w323 -> [w366]
                tunnel: [w364] -> w321
                tunnel: [w368] -> w320
                tunnel: [w367] -> w319
                tunnel: w322 -> [w367]
                tunnel: [w373] -> w318
                tunnel: w321 -> [w373]
                tunnel: w320 -> [_]
                tunnel: w319 -> [w379]
                tunnel: w317 -> [_]
                tunnel: [w375] -> w316
                tunnel: w309 -> [w378]
                tunnel: w308 -> [w377]
                tunnel: w315 -> [w376]
                tunnel: [w374] -> w313
                tunnel: [w372] -> w306
                frame #0 {
                  n243 = Negate(x=w339) -> (-x=w337:dbl)
                  n244 = local write "X Step Size (in)"(w337) -> ()
                  n245 = local write "Y Step Size (in)"(w335) -> ()
                  n246 = local write "Done Mov?"(FALSE ("Done Moving?")) -> ()
                }
                frame #1 {
                  n247 = property on="Move X (in)" class="Bool (strict)"("Val(Sgnl)"=w343) -> (error out=w342:errorcluster)  [unwired: 2 in, 1 out]
                }
                frame #2 {
                  n248 = while {
                    tunnel: [w352] -> w348
                    tunnel: w347 -> [_]
                    stop <- w354 stop-if-true
                    n249 = local read "Done Mov?"() -> (w352:bool)
                    n250 = local read "Abort"() -> (w353:bool)
                    n251 = Or(x=w353, y=w352) -> (x .or. y?=w354:bool)
                  }
                }
                frame #3 {
                  n252 = local write "Done Mov?"(FALSE ("Done Mov?")) -> ()
                  n253 = property on="Move Y (in)" class="Bool (strict)"("Val(Sgnl)"=TRUE) -> ()  [unwired: 2 in, 2 out]
                  n254 = Multiply(x=w361, y=w359) -> (x*y=w357:dbl)
                  n255 = Increment(x=w359) -> (x+1=w358:i32)
                  n256 = Divide(x=w357, y=w356) -> (x/y=w355:dbl)
                  n257 = Less Or Equal?(x=w356, y=w357) -> (x <= y?=w363:bool)
                }
                frame #4 {
                  n258 = while {
                    tunnel: [w370] -> w368
                    tunnel: [w369] -> w365
                    stop <- w371 stop-if-true
                    n259 = local read "Done Mov?"() -> (w370:bool)
                    n260 = local read "Abort"() -> (w369:bool)
                    n261 = Or(x=w370, y=w369) -> (x .or. y?=w371:bool)
                  }
                  n262 = Or(x=w366, y=w365) -> (x .or. y?=w364:bool)
                }
                frame #5 {
                  n263 = case shown="False" w373 {
                    tunnel: w379 -> [w386 _]
                    tunnel: w378 -> [w385 w388]
                    tunnel: w377 -> [w384 _]
                    tunnel: w376 -> [w383 w387]
                    tunnel: [w382 w388] -> w375
                    tunnel: [w381 w387] -> w374
                    frame False {
                      n264 = call "Measure and Update Array.vi"("Array In"=w385, "number of samples per channel"=w384, "task/channels in"=w383, "Row"=0, "Column"=w386) -> ("Array Out"=w382:dbl[][], "task out"=w381:refnum<k21>)  [unwired: 7 in, 2 out]
                      n265 = local write "Graph"(w382) -> ()
                    }
                    frame True {
                    }
                  }
                  n266 = Tick Count (ms)() -> (millisecond timer value=w372:u32)
                }
              }
            }
            frame True {
              n267 = Tick Count (ms)() -> (millisecond timer value=w390:u32)
            }
          }
          n268 = Tick Count (ms)() -> (millisecond timer value=w286:u32)
          n269 = Subtract(x=1.0, y=w279) -> (x-y=w281:dbl)
          n270 = Subtract(x=w285, y=w286) -> (x-y=w284:u32)
          n271 = Multiply(x=w284, y=w281) -> (x*y=w283:dbl)
          n272 = Multiply(x=w283, y=w282) -> (x*y=w276:dbl)
          n273 = Divide(x=w276, y=60000.0) -> (x/y=→"Time Left":dbl)
        }
        n274 = local write "array of values"(w268) -> ()
        n275 = flat-sequence {
          tunnel: w267 -> [w273]
          frame #0 {
            n276 = local write "Done Mov?"(FALSE) -> ()
            n277 = Wait (ms)(milliseconds to wait=u32 2000) -> ()  [unwired: 1 out]
            "(X,Y)" <- w273
          }
        }
        n278 = call <vilib>:"DAQmx Clear Task.vi"("task in"=w265) -> ()  [unwired: 14 in, 1 out]
      }
      frame "Flyover Scan" {
        # "Correction\nFactor"
        n279 = local read "Y Step Size"() -> (w465:dbl)
        n280 = local read "Y Length"() -> (w464:dbl)
        n281 = local read "X Length"() -> (w455:dbl)
        n282 = local read "Velocity"() -> (w458:dbl)
        n283 = local read "number of samples"() -> (w463:i32)
        n284 = local read "Measures/Pixel"() -> (w462:dbl)
        n285 = Multiply(x=w463, y=w462) -> (x*y=w461:dbl)
        n286 = Divide(x=w464, y=w465) -> (x/y=w452:dbl)
        n287 = local read "rate"() -> (w460:dbl)
        n288 = Divide(x=w461, y=w460) -> (x/y=w459:dbl)
        n289 = Round Toward +Infinity(x=w452) -> (ceil(x): smallest int >= x=w451:dbl)
        n290 = Multiply(x=w459, y=w458) -> (x*y=w454:dbl)
        n291 = Divide(x=w455, y=w454) -> (x/y=w457:dbl)
        n292 = Divide(x=w457, y=1.0) -> (x/y=w456:dbl)
        n293 = Initialize Array(-inf, w456, w451) -> (w468:dbl[][])
        n294 = local read "task out"() -> (w467:refnum<k21>)
        n295 = while {
          shift-right: [w479] -> _
          shift-left: w468 -> [w507]
          tunnel: w465 -> [w481]
          tunnel: w464 -> [w482]
          tunnel: w467 -> [w500]
          tunnel: [w499] -> w466
          tunnel: w462 -> [w498]
          tunnel: w463 -> [w497]
          tunnel: w451 -> [w477]
          i -> [w503]
          stop <- w486 stop-if-true
          n296 = Tick Count (ms)() -> (millisecond timer value=w476:u32)
          n297 = local write "Y Step Size (in)"(w481) -> ()
          n298 = flat-sequence {
            tunnel: [w536] -> w508
            tunnel: w507 -> [w536]
            tunnel: [w535] -> w505
            tunnel: w503 -> [w535]
            tunnel: [w546] -> w509
            tunnel: w508 -> [w546]
            tunnel: [w544] -> w506
            tunnel: w505 -> [w544]
            tunnel: [w541] -> w504
            tunnel: [w540] -> w501
            tunnel: w500 -> [w539]
            tunnel: [w556] -> w511
            tunnel: [w550] -> w510
            tunnel: w509 -> [w553]
            tunnel: w506 -> [w547]
            tunnel: w504 -> [w555]
            tunnel: w501 -> [w554]
            tunnel: w498 -> [w552]
            tunnel: w497 -> [w551]
            tunnel: [w548] -> w489
            tunnel: w511 -> [w584]
            tunnel: w510 -> [w581]
            tunnel: [w578] -> w480
            tunnel: [w583] -> w499
            tunnel: w489 -> [w579]
            tunnel: [w577] -> w475
            frame #0 {
              n299 = local read "X Length"() -> (w537:dbl)
              n300 = local write "X Step Size (in)"(w537) -> ()
              n301 = local write "Done Mov?"(FALSE ("Done Moving?")) -> ()
              n302 = Wait (ms)(milliseconds to wait=u32 50) -> ()  [unwired: 1 out]
            }
            frame #1 {
              n303 = property on="Move X (in)" class="Bool (strict)"("Val(Sgnl)"=TRUE ("Value (Signaling)")) -> ()  [unwired: 2 in, 2 out]
              n304 = call <vilib>:"DAQmx Start Task.vi"("task/channels in"=w539) -> ("task out"=w540:refnum<k21>)  [unwired: 13 in, 1 out]
              n305 = Initialize Array(-inf, 1 ("dimension size")) -> (w541:dbl[])
            }
            frame #2 {
              n306 = while {
                tunnel: [w566] -> w556
                shift-right: [w560] -> _
                shift-left: w555 -> [w564]
                tunnel: w554 -> [w562]
                tunnel: [w560] -> w549
                tunnel: w552 -> [w559]
                tunnel: w551 -> [w558]
                i -> [w561]
                stop <- w557 stop-if-true
                n307 = while {
                  tunnel: w558 -> [w571]
                  tunnel: w562 -> [w574]
                  tunnel: [w573] -> w566
                  tunnel: w559 -> [w568]
                  tunnel: [w567] -> w565 mode=indexing
                  i -> [w570]
                  stop <- w576 stop-if-true
                  n308 = local read "Abort"() -> (w575:bool)
                  n309 = Greater?(x=w570, y=w568) -> (0:w569:bool)
                  n310 = Or(x=w569, y=w575) -> (x .or. y?=w576:bool)
                  n311 = call-poly <vilib>:"DAQmx Read.vi"("task/channels in"=w574, "number of samples per channel"=w571) -> ("task out"=w573:refnum<k21>, "data"=w572:dbl[])  [unwired: 11 in, 1 out]
                  n312 = call-poly <vilib>:"Mean.vi"("X"=w572) -> ("mean"=w567:dbl)  [unwired: 1 out]
                }
                n313 = local read "Done Mov?"() -> (w557:bool)
                n314 = call-poly <vilib>:"Mean.vi"("X"=w565) -> ("mean"=w563:dbl)  [unwired: 1 out]
                n315 = Insert Into Array(array=w564, index=w561, new element=w563) -> (w560:dbl[])
                n316 = local write "Line Scan"(w560) -> ()
              }
              n317 = Insert Into Array(array=w553, index (col)=w547, new element=w549) -> (w550:dbl[][])  [unwired: 1 in]
              n318 = local write "array of values"(w550) -> ()
              n319 = local write "Graph"(w550) -> ()
              n320 = Array Size(array=w549) -> (size(s)=w548:i32)
            }
            frame #3 {
              n321 = local read "Abort"() -> (w577:bool)
              n322 = call <vilib>:"DAQmx Stop Task.vi"("task/channels in"=w584) -> ("task out"=w583:refnum<k21>)  [unwired: 13 in, 1 out]
              n323 = case shown="False" w577 {
                tunnel: w581 -> [w594 w595]
                tunnel: 0 -> [w593 _]
                tunnel: w579 -> [w592 _]
                tunnel: [w591 w595] -> w578
                frame False {
                  n324 = Array Subset(array=w594, index (row)=w593, length (row)=w592) -> (w591:dbl[][])  [unwired: 2 in]
                }
                frame True {
                }
              }
              n325 = Array Size(array=w578) -> (size(s)=w587:i32[])
              n326 = Index Array(array=w587, index=0) -> (element=w585:i32)
              n327 = local read "X=T,Y=F"() -> (w589:bool)
              n328 = case shown="True" w589 {
                tunnel: [w596 w597] -> w588
                frame False {
                  n329 = local read "Y Length"() -> (w596:dbl)
                }
                frame True {
                  n330 = local read "X Length"() -> (w597:dbl)
                }
              }
              n331 = Divide(x=w588, y=w585) -> (x/y=w582:dbl)
              n332 = property on="Graph" class="IntGraph (strict)"("XScale.Multiplier"=w582) -> ()  [unwired: 2 in, 2 out]
              n333 = local write "Done Mov?"(FALSE ("Done Mov?")) -> ()
              n334 = local write "X Step Size"(w582) -> ()
            }
          }
          n335 = Multiply(x=w503, y=w481) -> (x*y=w488:dbl)
          n336 = local read "Velocity"() -> (w487:dbl)
          n337 = Greater Or Equal?(x=w488, y=w482) -> (x >= y?=w502:bool)
          n338 = Divide(x=w488, y=w482) -> (x/y=w496:dbl)
          n339 = Subtract(x=1.0, y=w496) -> (x-y=w491:dbl)
          n340 = Divide(x=w491, y=60000.0) -> (x/y=w485:dbl)
          n341 = Divide(x=w482, y=w481) -> (x/y=w483:dbl)
          n342 = Multiply(x=w485, y=w483) -> (x*y=w484:dbl)
          n343 = Or(x=w502, y=w475) -> (x .or. y?=w486:bool)
          n344 = Array Subset(array=w480, index (col)=0, length (col)=w477) -> (w479:dbl[][])  [unwired: 2 in]
          n345 = case shown="False" w486 {
            tunnel: w479 -> [_ _]
            tunnel: [w514 u32 0 ("millisecond timer value")] -> w494
            tunnel: w487 -> [w512 _]
            frame False {
              w513 = 2.0 ("Velocity")
              n346 = flat-sequence {
                tunnel: w513 -> [_]
                tunnel: [w529] -> w514
                tunnel: w512 -> [w531]
                frame #0 {
                  n347 = property on="Set Vel/Acc" class="Bool (strict)"("Val(Sgnl)"=TRUE ("Value (Signaling)")) -> ()  [unwired: 2 in, 2 out]
                }
                frame #1 {
                  n348 = Wait (ms)(milliseconds to wait=u32 50) -> ()  [unwired: 1 out]
                }
                frame #2 {
                  n349 = local read "X Length"() -> (w519:dbl)
                  n350 = local write "Done Mov?"(FALSE ("Done Mov?")) -> ()
                  n351 = Negate(x=w519) -> (-x=w518:dbl)
                  n352 = local write "X Step Size (in)"(w518) -> ()
                }
                frame #3 {
                  n353 = property on="Move X (in)" class="Bool (strict)"("Val(Sgnl)"=TRUE ("Value (Signaling)")) -> ()  [unwired: 2 in, 2 out]
                }
                frame #4 {
                  n354 = while {
                    stop <- w523 stop-if-true
                    n355 = local read "Abort"() -> (w521:bool)
                    n356 = local read "Done Mov?"() -> (w522:bool)
                    n357 = Or(x=w522, y=w521) -> (x .or. y?=w523:bool)
                  }
                }
                frame #5 {
                  n358 = local write "Done Mov?"(FALSE ("Done Mov?")) -> ()
                }
                frame #6 {
                  n359 = property on="Move Y (in)" class="Bool (strict)"("Val(Sgnl)"=TRUE ("Value (Signaling)")) -> ()  [unwired: 2 in, 2 out]
                }
                frame #7 {
                  n360 = while {
                    stop <- w528 stop-if-true
                    n361 = local read "Abort"() -> (w526:bool)
                    n362 = local read "Done Mov?"() -> (w527:bool)
                    n363 = Or(x=w527, y=w526) -> (x .or. y?=w528:bool)
                  }
                }
                frame #8 {
                  n364 = local write "Done Mov?"(FALSE ("Done Mov?")) -> ()
                  n365 = Tick Count (ms)() -> (millisecond timer value=w529:u32)
                }
                frame #9 {
                  n366 = local write "Velocity"(w531) -> ()
                }
                frame #10 {
                  n367 = property on="Set Vel/Acc" class="Bool (strict)"("Val(Sgnl)"=TRUE) -> ()  [unwired: 2 in, 2 out]
                }
              }
              n368 = local write "Velocity"(w513) -> ()
            }
            frame True {
            }
          }
          n369 = Subtract(x=w494, y=w476) -> (x-y=w493:u32)
          n370 = Multiply(x=w493, y=w484) -> (x*y=w492:dbl)
          n371 = local write "Time Left"(w492) -> ()
        }
        n372 = flat-sequence {
          tunnel: ["Move to Origin" ("Scan Type")] -> w471
          tunnel: w466 -> [w473]
          frame #0 {
            n373 = Wait (ms)(milliseconds to wait=u32 2000) -> ()  [unwired: 1 out]
            n374 = call <vilib>:"DAQmx Clear Task.vi"("task in"=w473) -> ()  [unwired: 14 in, 1 out]
          }
        }
      }
      frame "Estimate X Step Size" {
        # "Correction Factor"
        n375 = local read "number of samples"() -> (w608:i32)
        n376 = local read "Measures/Pixel"() -> (w607:dbl)
        n377 = local read "Velocity"() -> (w604:dbl)
        n378 = Multiply(x=w608, y=w607) -> (x*y=w605:dbl)
        n379 = local read "rate"() -> (w606:dbl)
        n380 = Divide(x=w605, y=w606) -> (x/y=w603:dbl)
        n381 = Multiply(x=w604, y=w603) -> (x*y=w602:dbl)
        n382 = Multiply(x=w602, y=1.0 ("x*y")) -> (x*y=w601:dbl)
        n383 = local write "X Step Size"(w601) -> ()
      }
      frame "Line Scan" {
        n384 = local read "X=T,Y=F"() -> (w613:bool)
        n385 = local read "X Step Size"() -> (w609:dbl)
        n386 = case shown="False" w613 {
          tunnel: [w617 w618] -> w612
          frame False {
            n387 = local read "Y Step Size"() -> (w616:dbl)
            n388 = local read "Y Line Scan"() -> (w617:dbl[])
            n389 = local write "Y Step Size (in)"(w616) -> ()
          }
          frame True {
            n390 = local read "X Line Scan"() -> (w618:dbl[])
          }
        }
        n391 = local read "X Length"() -> (w611:dbl)
        n392 = local write "X Step Size (in)"(w609) -> ()
        n393 = while {
          tunnel: w613 -> [w632]
          shift-right: [w619] -> _
          shift-left: w612 -> [w625]
          tunnel: w611 -> [w622]
          tunnel: w609 -> [w621]
          tunnel: [w620] -> w610
          i -> [w631]
          stop <- w628 stop-if-true
          n394 = flat-sequence {
            tunnel: w632 -> [w638]
            tunnel: w631 -> [w635]
            tunnel: [w637] -> w630
            tunnel: [w636] -> w626
            tunnel: w625 -> [w636]
            tunnel: [w635] -> w623
            tunnel: w622 -> [w634]
            tunnel: w621 -> [w633]
            tunnel: w630 -> [w656]
            tunnel: [w655] -> w629
            tunnel: [w654] -> w627
            tunnel: w626 -> [w654]
            tunnel: [w653] -> w624
            tunnel: w623 -> [w653]
            tunnel: [w667] -> w628
            tunnel: w629 -> [w667]
            tunnel: w627 -> [w664]
            tunnel: [w663] -> w619
            tunnel: w624 -> [w662]
            tunnel: [w660] -> w620
            frame #0 {
              n395 = case shown="False" w638 {
                tunnel: w635 -> [w643 w648]
                tunnel: [w640 w649] -> w637
                tunnel: w634 -> [_ w647]
                tunnel: w633 -> [_ w646]
                frame False {
                  n396 = local read "Y Step Size (in)"() -> (w639:dbl)
                  n397 = local read "Y Length"() -> (w641:dbl)
                  n398 = Increment(x=w643) -> (x+1=w644:i32)
                  n399 = property on="Move Y (in)" class="Bool (strict)"("Val(Sgnl)"=TRUE ("Value (Signaling)")) -> ()  [unwired: 2 in, 2 out]
                  n400 = Multiply(x=w644, y=w639) -> (x*y=w642:dbl)
                  n401 = Less Or Equal?(x=w641, y=w642) -> (x <= y?=w640:bool)
                }
                frame True {
                  n402 = property on="Move X (in)" class="Bool (strict)"("Val(Sgnl)"=TRUE ("Value (Signaling)")) -> ()  [unwired: 2 in, 2 out]
                  n403 = Multiply(x=w648, y=w646) -> (x*y=w650:dbl)
                  n404 = Less Or Equal?(x=w647, y=w650) -> (x <= y?=w649:bool)
                }
              }
            }
            frame #1 {
              n405 = while {
                tunnel: [w657] -> w652
                stop <- w659 stop-if-true
                n406 = local read "Abort"() -> (w657:bool)
                n407 = local read "Done Mov?"() -> (w658:bool)
                n408 = Or(x=w658, y=w657) -> (x .or. y?=w659:bool)
              }
              n409 = Or(x=w656, y=w652) -> (x .or. y?=w655:bool)
            }
            frame #2 {
              n410 = local read "number of samples"() -> (w665:i32)
              n411 = local read "task out"() -> (w666:refnum<k21>)
              n412 = local write "Done Mov?"(FALSE ("Done Moving?")) -> ()
              n413 = call "Measure Line Scan.vi"("number of samples per channel"=w665, "Iterator"=w662, "task/channels in"=w666, "Array in"=w664) -> ("task out"=w660:refnum<k21>, "Array out"=w663:dbl[])  [unwired: 4 in, 2 out]
            }
          }
          n414 = local write "Line Scan"(w619) -> ()
        }
        n415 = call <vilib>:"DAQmx Clear Task.vi"("task in"=w610) -> ()  [unwired: 14 in, 1 out]
      }
      frame "Flyover Linescan" {
        n416 = flat-sequence {
          tunnel: [w680] -> w672
          tunnel: [w685] -> w673
          tunnel: w672 -> [w686]
          tunnel: [w682] -> w670
          tunnel: w674 -> [w694]
          tunnel: w673 -> [w693]
          tunnel: "Measures/Pixel" -> [w691]
          tunnel: w670 -> [w690]
          tunnel: [w692] -> w669
          tunnel: [w689] -> w668
          tunnel: w669 -> [w723]
          tunnel: w668 -> [w721]
          frame #0 {
            n417 = local read "X Length"() -> (w679:dbl)
            n418 = local read "Y Length"() -> (w677:dbl)
            n419 = local write "Done Mov?"(FALSE ("Done Moving?")) -> ()
            n420 = local write "X Step Size (in)"(w679) -> ()
            n421 = local write "Y Step Size (in)"(w677) -> ()
            n422 = local read "task out"() -> (w680:refnum<k21>)
          }
          frame #1 {
            n423 = local read "X=T,Y=F"() -> (w684:bool)
            n424 = call <vilib>:"DAQmx Start Task.vi"("task/channels in"=w686) -> ("task out"=w685:refnum<k21>)  [unwired: 13 in, 1 out]
            n425 = case shown="False" w684 {
              frame False {
                n426 = property on="Move Y (in)" class="Bool (strict)"("Val(Sgnl)"=TRUE ("Value (Signaling)")) -> ()  [unwired: 2 in, 2 out]
              }
              frame True {
                n427 = property on="Move X (in)" class="Bool (strict)"("Val(Sgnl)"=TRUE ("Value (Signaling)")) -> ()  [unwired: 2 in, 2 out]
              }
            }
            n428 = Initialize Array(-inf, 1 ("dimension size")) -> (w682:dbl[])
          }
          frame #2 {
            n429 = while {
              tunnel: w694 -> [w706]
              tunnel: w693 -> [w705]
              tunnel: [w704] -> w692
              tunnel: w691 -> [w700]
              shift-right: [w697] -> w689
              shift-left: w690 -> [w699]
              i -> [w698]
              stop <- w701 stop-if-true
              n430 = while {
                tunnel: w706 -> [w711]
                tunnel: w705 -> [w714]
                tunnel: [w713] -> w704
                tunnel: w700 -> [w708]
                tunnel: [w707] -> w696 mode=indexing
                i -> [w710]
                stop <- w716 stop-if-true
                n431 = local read "Abort"() -> (w715:bool)
                n432 = Greater?(x=w710, y=w708) -> (0:w709:bool)
                n433 = Or(x=w709, y=w715) -> (x .or. y?=w716:bool)
                n434 = call-poly <vilib>:"DAQmx Read.vi"("task/channels in"=w714, "number of samples per channel"=w711) -> ("task out"=w713:refnum<k21>, "data"=w712:dbl[])  [unwired: 11 in, 1 out]
                n435 = call-poly <vilib>:"Mean.vi"("X"=w712) -> ("mean"=w707:dbl)  [unwired: 1 out]
              }
              n436 = local read "Abort"() -> (w703:bool)
              n437 = local read "Done Mov?"() -> (w702:bool)
              n438 = Or(x=w702, y=w703) -> (x .or. y?=w701:bool)
              n439 = call-poly <vilib>:"Mean.vi"("X"=w696) -> ("mean"=w695:dbl)  [unwired: 1 out]
              n440 = Insert Into Array(array=w699, index=w698, new element=w695) -> (w697:dbl[])
              n441 = local write "Line Scan"(w697) -> ()
            }
          }
          frame #3 {
            n442 = Array Size(array=w721) -> (size(s)=w720:i32)
            n443 = local read "X=T,Y=F"() -> (w718:bool)
            n444 = call <vilib>:"DAQmx Stop Task.vi"("task/channels in"=w723) -> ("task out"=w724:refnum<k21>)  [unwired: 13 in, 1 out]
            n445 = local write "Done Mov?"(FALSE ("Done Mov?")) -> ()
            n446 = case shown="False" w718 {
              tunnel: [w725 w726] -> w717
              frame False {
                n447 = local read "Y Length"() -> (w725:dbl)
              }
              frame True {
                n448 = local read "X Length"() -> (w726:dbl)
              }
            }
            n449 = Divide(x=w717, y=w720) -> (x/y=w719:dbl)
            n450 = call <vilib>:"DAQmx Clear Task.vi"("task in"=w724) -> ()  [unwired: 14 in, 1 out]
            n451 = property on="Line Scan" class="WFGraph (strict)"("XScale.Multiplier"=w719) -> ()  [unwired: 2 in, 2 out]
          }
        }
        n452 = local read "number of samples"() -> (w674:i32)
      }
      frame "Move to Origin" {
        n453 = local read "Acceleration"() -> (w735:dbl)
        n454 = local read "Velocity"() -> (w736:dbl)
        n455 = flat-sequence {
          tunnel: w737 -> [_]
          tunnel: w729 -> [w753]
          tunnel: w728 -> [w752]
          frame #0 {
            n456 = while {
              stop <- w751 stop-if-true
              n457 = local read "Done Mov?"() -> (w751:bool)
              n458 = Wait (ms)(milliseconds to wait=u32 10) -> ()  [unwired: 1 out]
            }
          }
          frame #1 {
            n459 = local write "Done Mov?"(FALSE ("Done Mov?")) -> ()
            n460 = local write "Acceleration"(w752) -> ()
            n461 = local write "Velocity"(w753) -> ()
          }
          frame #2 {
            n462 = property on="Set Vel/Acc" class="Bool (strict)"("Val(Sgnl)"=TRUE ("Value (Signaling)")) -> ()  [unwired: 2 in, 2 out]
          }
          frame #3 {
            n463 = Wait (ms)(milliseconds to wait=u32 150) -> ()  [unwired: 1 out]
          }
        }
        n464 = flat-sequence {
          tunnel: w730 -> [w758]
          tunnel: [w758] -> w729
          tunnel: [w757] -> w728
          tunnel: w727 -> [w757]
          tunnel: [w773] -> w737
          frame #0 {
            n465 = property on="Read Position" class="Bool (strict)"("Val(Sgnl)"=TRUE ("Value (Signaling)")) -> ()  [unwired: 2 in, 2 out]
            n466 = Wait (ms)(milliseconds to wait=u32 120) -> ()  [unwired: 1 out]
          }
          frame #1 {
            n467 = while {
              stop <- w761 stop-if-true
              n468 = local read "Read Position"() -> (w762:bool)
              n469 = Wait (ms)(milliseconds to wait=u32 10) -> ()  [unwired: 1 out]
              n470 = Not(x=w762) -> (.not. x?=w761:bool)
            }
          }
          frame #2 {
            n471 = local read "Y Origin"() -> (w768:dbl)
            n472 = local read "X Orign"() -> (w765:dbl)
            n473 = local read "Y Pos"() -> (w767:dbl)
            n474 = local read "X Pos"() -> (w764:dbl)
            n475 = Subtract(x=w768, y=w767) -> (x-y=w769:dbl)
            n476 = Subtract(x=w765, y=w764) -> (x-y=w766:dbl)
            n477 = local write "Y Step Size (in)"(w769) -> ()
            n478 = local write "X Step Size (in)"(w766) -> ()
          }
          frame #3 {
            n479 = local write "Done Mov?"(FALSE ("Done Mov?")) -> ()
            n480 = property on="Move X (in)" class="Bool (strict)"("Val(Sgnl)"=TRUE ("Value (Signaling)")) -> ()  [unwired: 2 in, 2 out]
          }
          frame #4 {
            n481 = while {
              stop <- w772 stop-if-true
              n482 = local read "Done Mov?"() -> (w772:bool)
            }
          }
          frame #5 {
            n483 = local write "Done Mov?"(FALSE ("Done Mov?")) -> ()
            n484 = property on="Move Y (in)" class="Bool (strict)"("Val(Sgnl)"=TRUE ("Value (Signaling)")) -> (error out=w773:errorcluster)  [unwired: 2 in, 1 out]
          }
        }
        n485 = flat-sequence {
          tunnel: w736 -> [w740]
          tunnel: w735 -> [w741]
          tunnel: [w741] -> w733
          tunnel: [w740] -> w731
          tunnel: [w745] -> w734
          tunnel: w733 -> [w745]
          tunnel: [w744] -> w732
          tunnel: w731 -> [w744]
          tunnel: [w748] -> w727
          tunnel: w734 -> [w748]
          tunnel: w732 -> [w747]
          tunnel: [w747] -> w730
          frame #0 {
            n486 = local write "Acceleration"(10.0 ("Acceleration")) -> ()
            n487 = local write "Velocity"(2.0 ("Velocity")) -> ()
          }
          frame #1 {
            n488 = property on="Set Vel/Acc" class="Bool (strict)"("Val(Sgnl)"=TRUE ("Value (Signaling)")) -> ()  [unwired: 2 in, 2 out]
          }
          frame #2 {
            n489 = Wait (ms)(milliseconds to wait=u32 150) -> ()  [unwired: 1 out]
          }
        }
      }
      frame "Move to Saved Position" {
        n490 = flat-sequence {
          tunnel: [w796] -> w776
          frame #0 {
            n491 = property on="Read Position" class="Bool (strict)"("Val(Sgnl)"=TRUE ("Value (Signaling)")) -> ()  [unwired: 2 in, 2 out]
            n492 = Wait (ms)(milliseconds to wait=u32 120) -> ()  [unwired: 1 out]
          }
          frame #1 {
            n493 = while {
              stop <- w784 stop-if-true
              n494 = local read "Read Position"() -> (w785:bool)
              n495 = Wait (ms)(milliseconds to wait=u32 10) -> ()  [unwired: 1 out]
              n496 = Not(x=w785) -> (.not. x?=w784:bool)
            }
          }
          frame #2 {
            n497 = local read "X Pos 1"() -> (w791:dbl)
            n498 = local read "Y Pos 1"() -> (w789:dbl)
            n499 = local read "X Pos"() -> (w792:dbl)
            n500 = local read "Y Pos"() -> (w788:dbl)
            n501 = Subtract(x=w791, y=w792) -> (x-y=w790:dbl)
            n502 = Subtract(x=w789, y=w788) -> (x-y=w787:dbl)
            n503 = local write "Y Step Size (in)"(w787) -> ()
            n504 = local write "X Step Size (in)"(w790) -> ()
          }
          frame #3 {
            n505 = local write "Done Mov?"(FALSE ("Done Mov?")) -> ()
            n506 = property on="Move X (in)" class="Bool (strict)"("Val(Sgnl)"=TRUE ("Value (Signaling)")) -> ()  [unwired: 2 in, 2 out]
          }
          frame #4 {
            n507 = while {
              stop <- w795 stop-if-true
              n508 = local read "Done Mov?"() -> (w795:bool)
            }
          }
          frame #5 {
            n509 = local write "Done Mov?"(FALSE ("Done Mov?")) -> ()
            n510 = property on="Move Y (in)" class="Bool (strict)"("Val(Sgnl)"=TRUE ("Value (Signaling)")) -> (error out=w796:errorcluster)  [unwired: 2 in, 1 out]
          }
        }
        n511 = flat-sequence {
          tunnel: w776 -> [_]
          frame #0 {
            n512 = while {
              stop <- w780 stop-if-true
              n513 = local read "Done Mov?"() -> (w780:bool)
              n514 = Wait (ms)(milliseconds to wait=u32 10) -> ()  [unwired: 1 out]
            }
          }
          frame #1 {
            n515 = local write "Done Mov?"(FALSE ("Done Mov?")) -> ()
          }
        }
      }
      frame "Move to Cursor" {
        n516 = flat-sequence {
          tunnel: w801 -> [_]
          tunnel: [w814] -> w805
          tunnel: w805 -> [w824]
          tunnel: [w825] -> w799
          tunnel: [w827] -> w800
          tunnel: w799 -> [w827]
          frame #0 {
            n517 = while {
              stop <- w812 stop-if-true
              n518 = local read "Read Position"() -> (w813:bool)
              n519 = Not(x=w813) -> (.not. x?=w812:bool)
              n520 = Wait (ms)(milliseconds to wait=u32 10) -> ()  [unwired: 1 out]
            }
          }
          frame #1 {
            n521 = property on="Graph" class="IntGraph (strict)"("Active Cursor"=u32 0) -> (error out=w815:errorcluster)  [unwired: 2 in, 1 out]
            n522 = property on="Graph" class="IntGraph (strict)"(error in=w815) -> ("Cursor.Cursor Position"=w814:T3)  [unwired: 1 in, 2 out]
          }
          frame #2 {
            n523 = Unbundle By Name(w824) -> ("Cursor X"=w823:dbl, "Cursor Y"=w818:dbl)
            n524 = local read "X Pos"() -> (w822:dbl)
            n525 = local read "Y Pos"() -> (w821:dbl)
            n526 = Subtract(x=w823, y=w822) -> (x-y=w820:dbl)
            n527 = Subtract(x=w818, y=w821) -> (x-y=w819:dbl)
            n528 = local write "X Step Size (in)"(w820) -> ()
            n529 = local write "Y Step Size (in)"(w819) -> ()
            n530 = local write "Done Mov?"(FALSE ("Done Mov?")) -> ()
          }
          frame #3 {
            n531 = property on="Move Y (in)" class="Bool (strict)"("Val(Sgnl)"=TRUE) -> (error out=w825:errorcluster)  [unwired: 2 in, 1 out]
          }
          frame #4 {
            n532 = while {
              stop <- w829 stop-if-true
              n533 = local read "Done Mov?"() -> (w829:bool)
              n534 = Wait (ms)(milliseconds to wait=u32 10 ("millisecond timer value")) -> ()  [unwired: 1 out]
            }
          }
        }
        n535 = property on="Read Position" class="Bool (strict)"("Val(Sgnl)"=TRUE) -> (error out=w801:errorcluster)  [unwired: 2 in, 1 out]
        n536 = flat-sequence {
          tunnel: w800 -> [_]
          frame #0 {
            n537 = local write "Done Mov?"(FALSE ("Done Mov?")) -> ()
            n538 = property on="Move X (in)" class="Bool (strict)"("Val(Sgnl)"=TRUE) -> ()  [unwired: 2 in, 2 out]
          }
          frame #1 {
            n539 = while {
              stop <- w808 stop-if-true
              n540 = local read "Done Mov?"() -> (w808:bool)
              n541 = Wait (ms)(milliseconds to wait=u32 10 ("millisecond timer value")) -> ()  [unwired: 1 out]
            }
          }
          frame #2 {
            n542 = local write "Done Mov?"(FALSE ("Done Mov?")) -> ()
          }
        }
      }
      frame "Move to" {
        n543 = flat-sequence {
          frame #0 {
            n544 = property on="Read Position" class="Bool (strict)"("Val(Sgnl)"=TRUE ("Value (Signaling)")) -> ()  [unwired: 2 in, 2 out]
          }
          frame #1 {
            n545 = while {
              stop <- w833 stop-if-true
              n546 = local read "Read Position"() -> (w835:bool)
              n547 = Wait (ms)(milliseconds to wait=u32 10) -> ()  [unwired: 1 out]
              n548 = Not(x=w835) -> (.not. x?=w833:bool)
            }
          }
          frame #2 {
            n549 = local read "X=T,Y=F"() -> (w837:bool)
            n550 = case shown="False" w837 {
              tunnel: [w839 w845] -> w836
              frame False {
                n551 = flat-sequence {
                  tunnel: [w843] -> w839
                  frame #0 {
                    n552 = local read "Y Pos"() -> (w841:dbl)
                    n553 = Subtract(x="Y Move", y=w841) -> (x-y=w840:dbl)
                    n554 = local write "Y Step Size (in)"(w840) -> ()
                  }
                  frame #1 {
                    n555 = property on="Move Y (in)" class="Bool (strict)"("Val(Sgnl)"=TRUE ("Value (Signaling)")) -> (error out=w843:errorcluster)  [unwired: 2 in, 1 out]
                  }
                }
              }
              frame True {
                n556 = flat-sequence {
                  tunnel: [w849] -> w845
                  frame #0 {
                    n557 = local read "X Pos"() -> (w848:dbl)
                    n558 = Subtract(x="X Move", y=w848) -> (x-y=w846:dbl)
                    n559 = local write "X Step Size (in)"(w846) -> ()
                  }
                  frame #1 {
                    n560 = property on="Move X (in)" class="Bool (strict)"("Val(Sgnl)"=TRUE ("Value (Signaling)")) -> (error out=w849:errorcluster)  [unwired: 2 in, 1 out]
                  }
                }
              }
            }
            n561 = while {
              tunnel: w836 -> [_]
              stop <- w838 stop-if-true
              n562 = local read "Done Mov?"() -> (w838:bool)
            }
          }
        }
      }
      frame "Update Vel/Acc" {
        n563 = flat-sequence {
          frame #0 {
            n564 = property on="Set Vel/Acc" class="Bool (strict)"("Val(Sgnl)"=TRUE ("Value (Signaling)")) -> ()  [unwired: 2 in, 2 out]
          }
          frame #1 {
            n565 = Wait (ms)(milliseconds to wait=u32 50) -> ()  [unwired: 1 out]
          }
        }
      }
      frame "Save Position" {
        n566 = flat-sequence {
          frame #0 {
            n567 = property on="Read Position" class="Bool (strict)"("Val(Sgnl)"=TRUE ("Value (Signaling)")) -> ()  [unwired: 2 in, 2 out]
          }
          frame #1 {
            n568 = while {
              stop <- w859 stop-if-true
              n569 = local read "Read Position"() -> (w860:bool)
              n570 = Wait (ms)(milliseconds to wait=u32 10) -> ()  [unwired: 1 out]
              n571 = Not(x=w860) -> (.not. x?=w859:bool)
            }
          }
          frame #2 {
            n572 = local read "X Pos"() -> (→"X Pos 1":dbl)
            n573 = local read "Y Pos"() -> (→"Y Pos 1":dbl)
          }
        }
      }
      frame "Save Image" {
        n574 = property on="Graph" class="IntGraph (strict)"("Active Cursor"=u32 0) -> (error out=w874:errorcluster)  [unwired: 2 in, 1 out]
        n575 = property on="Graph" class="IntGraph (strict)"(error in=w874, "Cursor.Visible"=FALSE) -> (error out=w868:errorcluster)  [unwired: 1 in, 1 out]
        n576 = property on="Graph" class="IntGraph (strict)"(error in=w868, "Cursor Palette Vis"=FALSE ("Cursor Legend Visible")) -> (error out=w863:errorcluster)  [unwired: 1 in, 1 out]
        n577 = invoke on="Graph" class="IntGraph (strict)" method="Get Image"(error in=w863, "image depth"=24 ("Image Depth")) -> (error out=w870:errorcluster, "image data"=w871:T4)  [unwired: 4 in, 4 out]
        n578 = call <vilib>:"Write PNG File.vi"("error in (no error)"=w870, "image data"=w871) -> ("error out"=w867:errorcluster)  [unwired: 8 in, 1 out]
        n579 = property on="Graph" class="IntGraph (strict)"(error in=w867, "Cursor.Visible"=TRUE) -> (error out=w866:errorcluster)  [unwired: 1 in, 1 out]
        n580 = property on="Graph" class="IntGraph (strict)"(error in=w866, "Cursor Palette Vis"=TRUE ("Cursor.Visible")) -> ()  [unwired: 1 in, 2 out]
      }
      frame "Save Line graph" {
        n581 = property on="Line Scan" class="WFGraph (strict)"("Active Cursor"=u32 0) -> (error out=w884:errorcluster)  [unwired: 2 in, 1 out]
        n582 = property on="Line Scan" class="WFGraph (strict)"(error in=w884, "Cursor.Visible"=FALSE) -> (error out=w885:errorcluster)  [unwired: 1 in, 1 out]
        n583 = property on="Line Scan" class="WFGraph (strict)"(error in=w885, "Cursor Palette Vis"=FALSE ("Cursor Legend Visible")) -> (error out=w886:errorcluster)  [unwired: 1 in, 1 out]
        n584 = invoke on="Line Scan" class="WFGraph (strict)" method="Get Image"(error in=w886, "image depth"=24 ("Image Depth")) -> (error out=w888:errorcluster, "image data"=w887:T4)  [unwired: 4 in, 4 out]
        n585 = call <vilib>:"Write PNG File.vi"("error in (no error)"=w888, "image data"=w887) -> ("error out"=w889:errorcluster)  [unwired: 8 in, 1 out]
        n586 = property on="Line Scan" class="WFGraph (strict)"(error in=w889, "Cursor.Visible"=TRUE) -> (error out=w890:errorcluster)  [unwired: 1 in, 1 out]
        n587 = property on="Line Scan" class="WFGraph (strict)"(error in=w890, "Cursor Palette Vis"=TRUE ("Cursor Legend Visible")) -> ()  [unwired: 1 in, 2 out]
      }
      frame "Stop" {
      }
    }
  }
  n588 = while {
    shift-right: [w896] -> _
    shift-left: "Idle" -> [w897]
    tunnel: w10 -> [_]
    tunnel: w9 -> [_]
    stop <- w895 stop-if-true
    n589 = case shown="\"Idle\", Default" w897 {
      tunnel: [w899 "Stop" "Idle"] -> w896
      tunnel: [FALSE TRUE FALSE] -> w895
      frame "Idle", Default {
        n590 = flat-sequence {
          frame #0 {
            w900 = FALSE
            n591 = local write "Move X (in)"(w900) -> ()
            n592 = local write "Move Y (in)"(w900) -> ()
            n593 = local write "Moving?"(w900) -> ()
            n594 = local write "Move X"(w900) -> ()
            n595 = local write "Move Y"(w900) -> ()
          }
        }
        n596 = event shown="[1] \"Stop\": Value Change" {
          selector: _ -> [_ _ _ _ _ _]
          dyn-events: _ -> [_ _ _ _ _ _]
          timeout: _ -> [_ _ _ _ w908 _]
          tunnel: ["Wait" "Stop" "Moving" "Moving" "Moving" "Moving"] -> w899
          tunnel: [_ _ _ _ w908 _] -> _
          event Timeout {
            n597 = event-data() -> ()  [unwired: 1 in, 3 out]
          }
          event "Stop": Value Change {
            n598 = event-data() -> ()  [unwired: 1 in, 6 out]
          }
          event "Move X (in)": Value Change {
            n599 = event-data() -> ()  [unwired: 1 in, 6 out]
            n600 = local write "X=T,Y=F"(TRUE) -> ()
          }
          event "Move X": Value Change {
            n601 = event-data() -> ()  [unwired: 1 in, 6 out]
            n602 = local write "X Step Size (in)"("X Step Size") -> ()
            n603 = local write "X=T,Y=F"(TRUE ("X=T,Y=F")) -> ()
          }
          event "Move Y": Value Change {
            n604 = event-data() -> ()  [unwired: 1 in, 6 out]
            n605 = local write "X=T,Y=F"(FALSE ("X=T,Y=F")) -> ()
            n606 = local write "Y Step Size (in)"("Y Step Size") -> ()
          }
          event "Move Y (in)": Value Change {
            n607 = event-data() -> ()  [unwired: 1 in, 6 out]
            n608 = local write "X=T,Y=F"(FALSE) -> ()
          }
        }
      }
      frame "Stop" {
      }
      frame "Moving" {
        n609 = flat-sequence {
          tunnel: [w924] -> w916
          tunnel: w916 -> [w932]
          frame #0 {
            n610 = property on="Moving?" class="Bool (strict)"("Val(Sgnl)"=TRUE) -> ()  [unwired: 2 in, 2 out]
          }
          frame #1 {
            n611 = Wait (ms)(milliseconds to wait=u32 15 ("millisecond timer value")) -> ()  [unwired: 1 out]
          }
          frame #2 {
            n612 = property on="Read Position" class="Bool (strict)"("Val(Sgnl)"=TRUE ("Value (Signaling)")) -> ()  [unwired: 2 in, 2 out]
          }
          frame #3 {
            n613 = while {
              stop <- w922 stop-if-true
              n614 = local read "Read Position"() -> (w923:bool)
              n615 = Not(x=w923) -> (.not. x?=w922:bool)
            }
          }
          frame #4 {
            n616 = local read "X=T,Y=F"() -> (w927:bool)
            n617 = case shown="False" w927 {
              tunnel: [w928 w930] -> w925
              tunnel: [w929 w931] -> w926
              frame False {
                n618 = local read "Y Step Size (in)"() -> (w928:dbl)
                n619 = local read "Y Pos"() -> (w929:dbl)
              }
              frame True {
                n620 = local read "X Step Size (in)"() -> (w930:dbl)
                n621 = local read "X Pos"() -> (w931:dbl)
              }
            }
            n622 = Add(x=w926, y=w925) -> (x+y=w924:dbl)
          }
          frame #5 {
            n623 = while {
              tunnel: w932 -> [w938]
              stop <- w934 stop-if-true
              n624 = flat-sequence {
                tunnel: [w944] -> w935
                frame #0 {
                  n625 = property on="Read Position" class="Bool (strict)"("Val(Sgnl)"=TRUE ("Value (Signaling)")) -> ()  [unwired: 2 in, 2 out]
                }
                frame #1 {
                  n626 = while {
                    stop <- w942 stop-if-true
                    n627 = local read "Read Position"() -> (w943:bool)
                    n628 = Not(x=w943) -> (.not. x?=w942:bool)
                  }
                }
                frame #2 {
                  n629 = local read "X=T,Y=F"() -> (w945:bool)
                  n630 = case shown="False" w945 {
                    tunnel: [w946 w947] -> w944
                    frame False {
                      n631 = local read "Y Pos"() -> (w946:dbl)
                    }
                    frame True {
                      n632 = local read "X Pos"() -> (w947:dbl)
                    }
                  }
                }
              }
              n633 = Subtract(x=w938, y=w935) -> (x-y=w937:dbl)
              n634 = Absolute Value(x=w937) -> (abs(x)=w933:dbl)
              n635 = Less Or Equal?(x=w933, y=0.0001) -> (x <= y?=w934:bool)
              n636 = flat-sequence {
                tunnel: w934 -> [w939]
                frame #0 {
                  n637 = local write "Done Mov?"(w939) -> ()
                  n638 = Wait (ms)(milliseconds to wait=u32 5) -> ()  [unwired: 1 out]
                }
              }
            }
          }
        }
      }
    }
  }
  n639 = while {
    shift-right: [w953] -> _
    shift-left: "Idle" -> [w954]
    tunnel: [w951] -> w6
    tunnel: w10 -> [w951]
    tunnel: [w950] -> w4
    tunnel: w9 -> [w950]
    tunnel: w12 -> [w949]
    tunnel: w11 -> [w948]
    tunnel: [w949] -> w5
    tunnel: [w948] -> w1
    stop <- w952 stop-if-true
    n640 = case shown="\"Moving\"" w954 {
      tunnel: [w956 "Wait" "Idle" "Idle" "Idle" "Idle"] -> w953
      tunnel: [FALSE TRUE FALSE FALSE FALSE FALSE] -> w952
      tunnel: w951 -> [_ _ w970 w997 w1032 w1063]
      tunnel: w950 -> [_ _ w969 w998 w1031 w1062]
      tunnel: w949 -> [_ _ w967 w999 w1030 w1061]
      tunnel: w948 -> [_ _ w966 w1000 w1029 w1060]
      frame "Idle", Default {
        # "Might not be necesarry"
        n641 = flat-sequence {
          frame #0 {
            w957 = FALSE
            n642 = local write "Read Position"(w957) -> ()
            n643 = local write "Moving?"(w957) -> ()
            n644 = local write "Set Vel/Acc"(w957) -> ()
          }
        }
        n645 = event shown="[5] \"Stop\": Value Change" {
          selector: _ -> [_ _ _ _ _ _]
          dyn-events: _ -> [_ _ _ _ _ _]
          timeout: _ -> [_ _ _ _ _ _]
          tunnel: ["Idle" "Moving" "Read Position" "Set Vel/Acc" "Stop Action" "Stop"] -> w956
          event Timeout {
            n646 = event-data() -> ()  [unwired: 1 in, 3 out]
          }
          event "Moving?": Value Change {
            n647 = event-data() -> ()  [unwired: 1 in, 6 out]
          }
          event "Read Position": Value Change {
            n648 = event-data() -> ()  [unwired: 1 in, 6 out]
          }
          event "Set Vel/Acc": Value Change {
            n649 = event-data() -> ()  [unwired: 1 in, 6 out]
          }
          event "Abort": Value Change {
            n650 = event-data() -> ()  [unwired: 1 in, 6 out]
          }
          event "Stop": Value Change {
            n651 = event-data() -> ()  [unwired: 1 in, 6 out]
          }
        }
      }
      frame "Stop" {
      }
      frame "Moving" {
        # "This is the case that tells a motor to move by \"Y Step Size (in)\" or \"X Step Size (in)\""
        n652 = case shown="True" "X=T,Y=F" {
          tunnel: w970 -> [_ w985]
          tunnel: w969 -> [w973 _]
          tunnel: w967 -> [_ w986]
          tunnel: w966 -> [w975 _]
          frame False {
            n653 = local read "Settings Y"() -> (w983:T1)
            n654 = Unbundle(w983) -> ("Initial Position"=w981:dbl, "Move Absolute/Relative Position"=w980:dbl, "Step Delay (ms)"=w979:u32, "Velocity (mm/s)"=w978:dbl, "Acceleration (mm/s^2)"=w977:dbl)  [unwired: 1 out]
            n655 = local read "Y Step Size (in)"() -> (w982:dbl)
            n656 = Bundle("Y Step Size (in)"=w982, "Initial Position"=w981, "Move Absolute/Relative Position"=w980, "Step Delay (ms)"=w979, "Velocity (mm/s)"=w978, "Acceleration (mm/s^2)"=w977) -> (w976:T5)  [unwired: 1 in]
            n657 = local write "Settings Y"(w976) -> ()
            n658 = call "ActionEngine M2.vi"("ChannelNumber"=2, "Settings"=w976, "SerialNumber"=w975, "KCubeStepperControl"=w973, "Action"=ActionEngineEnum."Step") -> ()  [unwired: 4 in, 2 out]
          }
          frame True {
            n659 = local read "Settings X"() -> (w996:T1)
            n660 = Unbundle(w996) -> ("Initial Position"=w995:dbl, "Move Absolute/Relative Position"=w994:dbl, "Step Delay (ms)"=w993:u32, "Velocity (mm/s)"=w992:dbl, "Acceleration (mm/s^2)"=w991:dbl)  [unwired: 1 out]
            n661 = local read "X Step Size (in)"() -> (w990:dbl)
            n662 = Bundle("X Step Size (in)"=w990, "Initial Position"=w995, "Move Absolute/Relative Position"=w994, "Step Delay (ms)"=w993, "Velocity (mm/s)"=w992, "Acceleration (mm/s^2)"=w991) -> (w987:T6)  [unwired: 1 in]
            n663 = local write "Settings X"(w987) -> ()
            n664 = call "ActionEngine M1.vi"("ChannelNumber"=1, "Settings"=w987, "SerialNumber"=w986, "KCubeStepperControl"=w985, "Action"=ActionEngineEnum."Step") -> ()  [unwired: 4 in, 2 out]
          }
        }
      }
      frame "Set Vel/Acc" {
        n665 = flat-sequence {
          tunnel: [w1006] -> w1002
          tunnel: [w1005] -> w1001
          tunnel: w1002 -> [w1028]
          tunnel: w1001 -> [w1027]
          tunnel: w1000 -> [w1024]
          tunnel: w999 -> [w1021]
          tunnel: w998 -> [w1020]
          tunnel: w997 -> [w1019]
          frame #0 {
            n666 = local read "Settings Y"() -> (w1017:T1)
            n667 = local read "Settings X"() -> (w1018:T1)
            n668 = local read "Acceleration"() -> (w1007:dbl)
            n669 = local read "Velocity"() -> (w1008:dbl)
            n670 = Unbundle(w1017) -> ("Step Size (mm)"=w1012:sgl, "Initial Position"=w1011:dbl, "Move Absolute/Relative Position"=w1010:dbl, "Step Delay (ms)"=w1009:u32)  [unwired: 2 out]
            n671 = Unbundle(w1018) -> ("Step Size (mm)"=w1016:sgl, "Initial Position"=w1015:dbl, "Move Absolute/Relative Position"=w1014:dbl, "Step Delay (ms)"=w1013:u32)  [unwired: 2 out]
            n672 = Bundle("Step Size (mm)"=w1016, "Initial Position"=w1015, "Move Absolute/Relative Position"=w1014, "Step Delay (ms)"=w1013, "Velocity"=w1008, "Acceleration"=w1007) -> (w1006:T7)  [unwired: 1 in]
            n673 = Bundle("Step Size (mm)"=w1012, "Initial Position"=w1011, "Move Absolute/Relative Position"=w1010, "Step Delay (ms)"=w1009, "Velocity"=w1008, "Acceleration"=w1007) -> (w1005:T7)  [unwired: 1 in]
            n674 = local write "Settings X"(w1006) -> ()
            n675 = local write "Settings Y"(w1005) -> ()
          }
          frame #1 {
            n676 = call "ActionEngine M1.vi"("ChannelNumber"=1, "Settings"=w1028, "SerialNumber"=w1021, "KCubeStepperControl"=w1019, "Action"=ActionEngineEnum."Settings") -> ()  [unwired: 4 in, 2 out]
            n677 = call "ActionEngine M2.vi"("ChannelNumber"=2, "Settings"=w1027, "SerialNumber"=w1024, "KCubeStepperControl"=w1020, "Action"=ActionEngineEnum."Settings") -> ()  [unwired: 4 in, 2 out]
          }
        }
      }
      frame "Stop Action" {
        n678 = local read "Flyover X Linescan"() -> (w1035:bool)
        n679 = local read "Flyover Y Linescan"() -> (w1034:bool)
        n680 = Compound Arithmetic op=OR(w1035, w1034) -> (w1033:bool)
        n681 = case shown="True" w1033 {
          tunnel: w1032 -> [_ w1041]
          tunnel: w1031 -> [_ w1040]
          tunnel: w1030 -> [_ w1039]
          tunnel: w1029 -> [_ w1038]
          frame False {
          }
          frame True {
            n682 = flat-sequence {
              tunnel: w1041 -> [w1047]
              tunnel: w1040 -> [w1046]
              tunnel: w1039 -> [w1043]
              tunnel: w1038 -> [w1042]
              frame #0 {
                n683 = local read "Settings X"() -> (w1045:T1)
                n684 = local read "Settings Y"() -> (w1044:T1)
                n685 = call "ActionEngine M1.vi"("Settings"=w1045, "SerialNumber"=w1043, "KCubeStepperControl"=w1047, "Action"=ActionEngineEnum."Stop Action") -> ()  [unwired: 5 in, 2 out]
                n686 = call "ActionEngine M2.vi"("Settings"=w1044, "SerialNumber"=w1042, "KCubeStepperControl"=w1046, "Action"=ActionEngineEnum."Stop Action") -> ()  [unwired: 5 in, 2 out]
              }
              frame #1 {
                n687 = local read "Y Length"() -> (w1059:dbl)
                n688 = local read "X Length"() -> (w1057:dbl)
                n689 = local read "Y Origin"() -> (w1051:dbl)
                n690 = local read "X Orign"() -> (w1054:dbl)
                n691 = Divide(x=w1057, y=2.0) -> (x/y=w1055:dbl)
                n692 = Divide(x=w1059, y=2.0) -> (x/y=w1052:dbl)
                n693 = Add(x=w1054, y=w1055) -> (x+y=w1053:dbl)
                n694 = Add(x=w1051, y=w1052) -> (x+y=w1050:dbl)
                n695 = local write "X Pos"(w1053) -> ()
                n696 = local write "Y Pos"(w1050) -> ()
              }
            }
          }
        }
      }
      frame "Read Position" {
        n697 = flat-sequence {
          tunnel: w1063 -> [w1071]
          tunnel: w1062 -> [w1070]
          tunnel: w1061 -> [w1067]
          tunnel: w1060 -> [w1066]
          frame #0 {
            n698 = local read "Settings Y"() -> (w1068:T1)
            n699 = local read "Settings X"() -> (w1069:T1)
            n700 = call "ActionEngine M2.vi"("Settings"=w1068, "SerialNumber"=w1066, "KCubeStepperControl"=w1070, "Action"=ActionEngineEnum."Get Position") -> ("Current Position"=w1072:dbl)  [unwired: 5 in, 1 out]
            n701 = call "ActionEngine M1.vi"("Settings"=w1069, "SerialNumber"=w1067, "KCubeStepperControl"=w1071, "Action"=ActionEngineEnum."Get Position") -> ("Current Position"=w1073:dbl)  [unwired: 5 in, 1 out]
            n702 = local write "Y Pos"(w1072) -> ()
            n703 = local write "X Pos"(w1073) -> ()
          }
          frame #1 {
            n704 = local write "Read Position"(FALSE) -> ()
          }
        }
      }
    }
  }
  n705 = flat-sequence {
    tunnel: w6 -> [w1083]
    tunnel: w5 -> [w1081]
    tunnel: w4 -> [w1079]
    tunnel: [w1079] -> w3
    tunnel: [w1078] -> w2
    tunnel: w1 -> [w1078]
    tunnel: w3 -> [w1088]
    tunnel: w2 -> [w1086]
    frame #0 {
      n706 = local read "Settings X"() -> (w1080:T1)
      n707 = call "ActionEngine M1.vi"("ChannelNumber"=1, "Settings"=w1080, "SerialNumber"=w1081, "KCubeStepperControl"=w1083, "Action"=ActionEngineEnum."Close Connection") -> ()  [unwired: 4 in, 2 out]
    }
    frame #1 {
      n708 = local read "Settings Y"() -> (w1085:T1)
      n709 = call "ActionEngine M2.vi"("ChannelNumber"=2, "Settings"=w1085, "SerialNumber"=w1086, "KCubeStepperControl"=w1088, "Action"=ActionEngineEnum."Close Connection") -> ()  [unwired: 4 in, 2 out]
    }
    frame #2 {
      n710 = local write "Stop"(FALSE ("Stop")) -> ()
    }
  }
